vi "WS1050 36 DUT Reliability HD_Cycling_CP CVSweep_Ver1.2.vi"() -> ()   [LabVIEW 2012]
uses:
  WS_VCAP Driver 029/Source/WSVCAP Shell/Type Defs/WSVCAP SHL I2C DUT Mask Mode Enum.ctl
  SubVI/WS105x Run Sequences.ctl
  <vilib>/Utility/file.llb/Read From Spreadsheet File (DBL).vi
panel:
  out "All Data Out":string[](array[string])
  in  "RFFE Slave Address":u8=7 caption="Slave Address" format="0x%02x"
  in  "Reg1_Bit Cntrl":string[](array[string])=["01", "02", "04", "08", "10", "20", "40", "80", "03", "06", "0C", "D8", "33", "66", "CC", "07", "0E", "1C", "38", "70", "E0", "0F", "1E", "3C", "78", "F0", "1F", "3E", "7C", "F8", "3F", "7E", "FC", "7F", "FE", "FD", "FB", "F7", "EF", "DF", "BF", "7F", "FC", "F9", "F3", "E7", "CF", "9F", "3F", "F8", "F1", "E3", "C7", "8F", "1F", "F0", "E1", "C3", "87", "0F", "E0", "C1", "83", "07", "C0", "81", "03", "AA", "55", "00"]
  in  "VPI_Cmd":string[](array[string])=["00", "3B", "00"]
  in  "VPI Name":string[](array[string])=["All_Drivers OFF", "All Drivers ON", "All Drivers OFF2"]
  in  "Tab Control":T1(tab)
  in  "CP with DVA ON":i32(ring) items=["CP HDC 35V", "CP HDC 40.25V", "CP HDC 27.5V", "CP HDC 30.5V", "CP HDC 44V", "CP HDC 50V", "CP HDC 55V", "CP HDC 42.5V", "CP HDC 32V"]
  in  "No of Cmd":i64=2
  in  "Board#":string="BRD5"
  in  "Serial Number":string[][](table)=[["DUT", "SN"], ["DUT1", "1"], ["DUT2", "2"], ["DUT3", "3"], ["DUT4", "4"], ["DUT5", "5"], ["DUT6", "6"], ["DUT7", "7"], ["DUT8", "8"], ["DUT9", "9"], ["DUT10", "10"], ["DUT11", "11"], ["DUT12", "12"], ["DUT13", "13"], ["DUT14", "14"], ["DUT15", "15"], ["DUT16", "16"], ["DUT17", "17"], ["DUT18", "18"], ["DUT19", "19"], ["DUT20", "20"], ["DUT21", "21"], ["DUT22", "22"], ["DUT23", "23"], ["DUT24", "24"], ["DUT25", "25"], ["DUT26", "26"], ["DUT27", "27"], ["DUT28", "28"], ["DUT29", "29"], ["DUT30", "30"], ["DUT31", "31"], ["DUT32", "32"], ["DUT33", "33"], ["DUT34", "34"], ["DUT35", "35"], ["DUT36", "36"]]
  in  "SPI Clock Rate (Hz)":dbl=5000000.0 caption="Cycle Speed" format="%.1p Hz"
  in  "Wafer#":string="T7-EB"
  in  "File Name":string="CYC_WS1050_T7_EB_65C_40V_25DC_BRD5_150911_1"
  in  "TMN DC\\CAP Data Log File Path":path=path "C:/WS1050 36 DUT Data"
  in  "Test Program":string="WS1050 36 DUT HD_Cycling_CP CV Sweep Ver1.2"
  out "Current Date":string="8/28/2014"
  out "Current Time":string="0950"
  in  "Start Date":string="10/21/2014"
  in  "Start Time":string="1542"
  in  "Comment":string="CYC65C40V"
  in  "OK Button":bool
  in  "Calibration":bool
  in  "Verify CP":bool
  in  "CP Setting":i32(ring) items=["CP OFF", "CP ON", "CP 35V", "CP 40V", "DVA ON", "DVA OFF", "REG1 ON", "REG1 OFF", "REG2 ON", "REG2 OFF", "REG3 ON", "REG3 OFF"]
  in  "Set VDD":dbl=3.7 format="%.3g"
  in  "Command":string[](array[string])=["0702013B3B3B", "070201000000", "0702013B0000"]
  in  "Clock Rate (Hz)":dbl=1000000.0 caption="Meas Speed" format="%.1p Hz"
  out "AR  Measurent(Hz)":dbl
  in  "PS1 Source":refnum<visa-resource-name>="GPIB0::5::INSTR"
  in  "Ke2000":refnum<visa-resource-name>="GPIB0::9::INSTR"
  in  "CP to HD/Cycle":i32(ring)=1 items=["CP HDC 35V", "CP HDC 40.25V", "CP HDC 27.5V", "CP HDC 30.5V", "CP HDC 44V", "CP HDC 50V", "CP HDC 55V", "CP HDC 42.5V", "CP HDC 32V"]
  out "Simulate FPGA":bool
  out "Online":bool
  out "AR Cycling(Hz)":dbl=5000000.0
  in  "Ke2400":refnum<visa-resource-name>="GPIB0::3::INSTR"
  in  "Initialize AD7747":bool
  in  "DUT Mask Mode":T2=enum."All"
  out "Activity Log":string="05/19/2014 -- 12:24:35.853::WSVCAP::APP::Application Started\n05/19/2014 -- 12:24:37.606::WSVCAP::WSVCAP SHL::WR I2C-REG:0x0A;MASK:0xFFFFFFFFFFFF;C1 DATA:22:22:22:22:22:22:22:22:22:22:22:22:22:22:22:22;C2 DATA:22:22:22:22:22:22:22:22:22:22:22:22:22:22:22:22;C3 DATA:22:22:22:22:22:22:22:22:22:22:22:22:22:22:22:22\r\n05/19/2014 -- 12:24:37.773::WSVCAP::WSVCAP SHL::WR I2C-ST:0,0,4,1\r\n05/19/2014 -- 12:24:37.903::WSVCAP::WSVCAP SHL::RD I2C-BYTES:4;ADD:0x00;MASK:0xFFFFFFFFFFFF\r\n05/19/2014 -- 12:24:38.045::WSVCAP::WSVCAP SHL::RD I2C:C1 DATA:2:2:2:2:2:2:2:2:2:2:2:2:2:2:2:2|A7:A9:AA:82:82:7F:82:81:82:81:83:82:81:82:82:81|46:36:BB:88:44:A3:E9:2B:32:20:ED:25:BB:3D:68:B|2C:6A:EB:A7:22:56:FE:CC:36:82:D7:B0:3B:48:F9:CC;C2 DATA:2:2:2:2:2:2:2:2:2:2:2:2:2:2:2:2|94:94:94:80:80:80:80:80:81:7E:7E:81:80:7E:80:80|47:33:15:82:62:B:E8:1C:D7:C3:7D:41:7C:B7:4C:2A|C4:B4:AE:8:1E:D1:4E:37:11:C0:6F:63:42:9D:63:B5;C3 DATA:2:2:2:2:2:2:2:2:2:2:2:2:2:2:2:2|95:95:95:81:81:7E:81:80:84:7D:80:83:81:7E:7F:80|AB:C4:14:B5:7B:52:DF:C9:79:5D:5F:30:99:31:1E:F4|6E:5C:F7:A8:C3:EB:7B:EF:33:92:89:77:4D:67:75:DD;STATUS:0:0:4:0\r\n05/19/2014 -- 12:24:38.046::WSVCAP::WSVCAP SHL::WR I2C-REG:0x0A;MASK:0xFFFFFFFFFFFF;C1 DATA:22:22:22:22:22:22:22:22:22:22:22:22:22:22:22:22;C2 DATA:22:22:22:22:22:22:22:22:22:22:22:22:22:22:22:22;C3 DATA:22:22:22:22:22:22:22:22:22:22:22:22:22:22:22:22\r\n05/19/2014 -- 12:24:38.089::WSVCAP::WSVCAP SHL::WR I2C-ST:0,0,4,1\r\n05/19/2014 -- 12:24:38.219::WSVCAP::WSVCAP SHL::RD I2C-BYTES:4;ADD:0x00;MASK:0xFFFFFFFFFFFF\r\n05/19/2014 -- 12:24:38.362::WSVCAP::WSVCAP SHL::RD I2C:C1 DATA:2:2:2:2:2:2:2:2:2:2:2:2:2:2:2:2|A7:AB:AA:82:82:82:83:83:82:82:82:82:7F:82:82:81|4B:32:96:83:3E:61:43:17:25:62:AB:4D:A2:40:2E:5|3C:76:2B:B4:EE:E4:A9:1A:AA:A:26:C7:21:2E:87:5B;C2 DATA:2:2:2:2:2:2:2:2:2:2:2:2:2:2:2:2|94:94:94:80:80:80:80:80:80:7F:80:81:80:80:7F:80|4A:32:19:7D:19:6C:79:46:61:7F:4B:B8:A5:30:F3:14|B4:70:A:8C:9C:DC:43:FA:1E:A:C6:21:A:A9:13:F3;C3 DATA:2:2:2:2:2:2:2:2:2:2:2:2:2:2:2:2|95:97:94:81:80:81:82:81:80:7E:81:84:7F:81:80:80|B2:32:D0:A7:9E:4C:AB:D4:EE:D9:F0:82:B7:91:7:FF|C1:91:B6:3D:D8:E:1B:4F:9F:6A:F1:6C:E7:3F:7:BA;STATUS:0:0:4:0\r\n05/19/2014 -- 12:24:38.364::WSVCAP::WSVCAP SHL::WR I2C-REG:0x0A;MASK:0xFFFFFFFFFFFF;C1 DATA:22:22:22:22:22:22:22:22:22:22:22:22:22:22:22:22;C2 DATA:22:22:22:22:22:22:22:22:22:22:22:22:22:22:22:22;C3 DATA:22:22:22:22:22:22:22:22:22:22:22:22:22:22:22:22\r\n05/19/2014 -- 12:24:38.406::WSVCAP::WSVCAP SHL::WR I2C-ST:0,0,4,1\r\n05/19/2014 -- 12:24:38.536::WSVCAP::WSVCAP SHL::RD I2C-BYTES:4;ADD:0x00;MASK:0xFFFFFFFFFFFF\r\n05/19/2014 -- 12:24:38.678::WSVCAP::WSVCAP SHL::RD I2C:C1 DATA:2:2:2:2:2:2:2:2:2:2:2:2:2:2:2:2|A7:A9:AB:82:82:81:82:82:82:82:82:82:82:82:82:81|46:71:4C:87:43:3D:7F:FC:25:4F:8E:54:97:3E:60:8C|AA:F4:1F:B5:CE:43:1F:36:9:87:9C:78:86:5:B6:8E;C2 DATA:2:2:2:2:2:2:2:2:2:2:2:2:2:2:2:2|94:94:94:80:7F:7F:80:80:80:80:80:81:80:80:80:80|49:36:18:7D:6E:C5:E4:3C:81:2E:41:D3:75:71:E3:72|E8:D3:E6:D1:E0:48:AE:D4:54:D:E8:8E:B4:41:68:4;C3 DATA:2:2:2:2:2:2:2:2:2:2:2:2:2:2:2:2|95:95:95:81:7F:7F:81:81:81:81:81:84:81:81:82:81|B3:F5:90:AB:82:69:7B:93:D0:77:E8:D5:E8:8C:84:E8|B9:AC:EE:2B:B6:71:8F:4A:74:31:56:BB:8A:B7:A0:C8;STATUS:0:0:4:0\r\n05/19/2014 -- 12:24:38.681::WSVCAP::WSVCAP SHL::WR I2C-REG:0x0A;MASK:0xFFFFFFFFFFFF;C1 DATA:22:22:22:22:22:22:22:22:22:22:22:22:22:22:22:22;C2 DATA:22:22:22:22:22:22:22:22:22:22:22:22:22:22:22:22;C3 DATA:22:22:22:22:22:22:22:22:22:22:22:22:22:22:22:22\r\n05/19/2014 -- 12:24:38.723::WSVCAP::WSVCAP SHL::WR I2C-ST:0,0,4,1\r\n05/19/2014 -- 12:24:38.854::WSVCAP::WSVCAP SHL::RD I2C-BYTES:4;ADD:0x00;MASK:0xFFFFFFFFFFFF\r\n05/19/2014 -- 12:24:38.996::WSVCAP::WSVCAP SHL::RD I2C:C1 DATA:2:2:2:2:2:2:2:2:2:2:2:2:2:2:2:2|A7:A9:AA:82:82:7F:83:81:82:81:84:82:7F:82:7F:82|43:FB:E:7F:3C:AD:35:35:26:A2:6C:21:4B:3D:8:6|63:9A:E1:F3:95:32:91:42:90:3C:78:1F:5C:D7:5F:D8;C2 DATA:2:2:2:2:2:2:2:2:2:2:2:2:2:2:2:2|94:94:94:80:80:80:80:80:81:80:7E:81:80:7E:7F:80|48:36:18:7F:5E:3D:69:83:DE:AE:A1:9E:31:AE:BB:96|15:A0:44:17:13:FD:CC:C8:6D:B2:EF:A7:C:C7:3B:F;C3 DATA:2:2:2:2:2:2:2:2:2:2:2:2:2:2:2:2|95:96:94:81:81:7E:82:80:84:80:80:84:7F:7E:7D:82|AD:3B:6D:A9:7C:57:9D:F5:7A:96:23:5C:36:2D:ED:5A|CD:46:DB:3B:C7:BD:70:60:33:B8:B:F7:63:A:51:4D;STATUS:0:0:4:0\r\n05/19/2014 -- 12:24:38.998::WSVCAP::WSVCAP SHL::WR I2C-REG:0x0A;MASK:0xFFFFFFFFFFFF;C1 DATA:22:22:22:22:22:22:22:22:22:22:22:22:22:22:22:22;C2 DATA:22:22:22:22:22:22:22:22:22:22:22:22:22:22:22:22;C3 DATA:22:22:22:22:22:22:22:22:22:22:22:22:22:22:22:22\r\n05/19/2014 -- 12:24:39.040::WSVCAP::WSVCAP SHL::WR I2C-ST:0,0,4,1\r\n05/19/2014 -- 12:24:39.170::WSVCAP::WSVCAP SHL::RD I2C-BYTES:4;ADD:0x00;MASK:0xFFFFFFFFFFFF\r\n05/19/2014 -- 12:24:39.311::WSVCAP::WSVCAP SHL::RD I2C:C1 DATA:2:2:2:2:2:2:2:2:2:2:2:2:2:2:2:2|A7:AA:AB:82:82:81:82:81:82:81:82:82:82:82:7F:82|44:F1:90:87:45:44:C8:2C:2C:F1:FC:1B:94:3B:3C:75|4A:49:95:19:99:73:64:3:23:24:F3:A2:5E:7F:C4:B6;C2 DATA:2:2:2:2:2:2:2:2:2:2:2:2:2:2:2:2|94:94:94:80:80:80:80:7F:80:80:7E:80:80:7E:7F:80|4C:36:17:7D:A8:9F:DE:C7:53:6D:8A:F4:41:A5:C6:E0|90:2E:24:C:D9:22:E4:76:3B:40:1D:53:33:B1:3E:4D;C3 DATA:2:2:2:2:2:2:2:2:2:2:2:2:2:2:2:2|95:97:95:81:81:7F:81:80:80:81:7F:82:81:7E:7D:82|AE:2B:A7:AB:CC:CD:A4:38:FD:17:80:F2:92:2D:45:C4|76:E5:D:B9:AD:B5:BA:8D:28:32:9E:42:B7:20:4A:D9;STATUS:0:0:4:0\r\n05/19/2014 -- 12:24:39.313::WSVCAP::WSVCAP SHL::WR I2C-REG:0x0A;MASK:0xFFFFFFFFFFFF;C1 DATA:22:22:22:22:22:22:22:22:22:22:22:22:22:22:22:22;C2 DATA:22:22:22:22:22:22:22:22:22:22:22:22:22:22:22:22;C3 DATA:22:22:22:22:22:22:22:22:22:22:22:22:22:22:22:22\r\n05/19/2014 -- 12:24:39.355::WSVCAP::WSVCAP SHL::WR I2C-ST:0,0,4,1\r\n05/19/2014 -- 12:24:39.486::WSVCAP::WSVCAP SHL::RD I2C-BYTES:4;ADD:0x00;MASK:0xFFFFFFFFFFFF\r\n05/19/2014 -- 12:24:39.628::WSVCAP::WSVCAP SHL::RD I2C:C1 DATA:2:2:2:2:2:2:2:2:2:2:2:2:2:2:2:2|A7:A9:AA:82:82:82:83:82:82:82:82:82:7F:82:7F:82|47:18:E4:87:3E:E7:6:65:25:92:37:38:A8:3E:89:85|7C:A7:7:2B:A3:7A:EC:EF:89:ED:F4:D3:D8:BC:3A:F5;C2 DATA:2:2:2:2:2:2:2:2:2:2:2:2:2:2:2:2|94:94:94:80:7F:80:80:7F:81:80:7E:80:80:80:81:80|49:37:17:80:76:25:6A:F8:DF:55:97:4D:B8:5B:2B:B1|13:E3:9A:3E:1A:2D:4F:B6:DB:E9:61:FA:8B:D6:9:CC;C3 DATA:2:2:2:2:2:2:2:2:2:2:2:2:2:2:2:2|95:95:95:81:7F:80:82:81:84:80:7F:81:80:81:7F:82|AF:93:3B:AF:5B:11:82:E4:7E:C3:2D:72:9:96:D9:A|DB:96:F2:10:5F:64:9A:C6:98:12:27:7D:10:D3:20:D9;STATUS:0:0:4:0\r\n05/19/2014 -- 12:24:40.132::WSVCAP::WSVCAP SHL::CLOSE\r\n"
  in  "C1 Cap DAC":u8=128 caption="B Data In" format="0x%02x"
  in  "C2 Cap DAC":u8=128 caption="B Data In" format="0x%02x"
  in  "C3 Cap DAC":u8=128 caption="B Data In" format="0x%02x"
  out "IDD Brd(uA)":string
  in  "Repeat Meas(s)":u32=900
  in  "Real No. From\nLookup Table":bool
  in  "Control Panel":T3={"Verify Socket"=FALSE, "HD/CYC"=FALSE, "E-CAL"=FALSE, "DVA"=FALSE, "VPI"=TRUE, "VSA"=TRUE, "HS"=FALSE}
  out "Verify Socket":bool
  out "HD/CYC":bool
  out "E-CAL":bool
  out "DVA":bool
  out "VPI":bool
  out "VSA":bool
  out "HS":bool
  in  "Lot#":string="WS1050"
  out "AD7747 Values":string[][](table)
  in  "Freq(Hz)":string="12K"
  in  "Reset P/S":bool
  in  "Test Sequences":i32(ring) items=["C1_C2_C3", "C2_C1_C3", "C3_C2_C1"]
  in  "WS1050/51":bool=TRUE
  in  "% Duty Cycle":string="25"
  in  "Cmd To HD":string="0702013B3B3B"
  in  "Post CMd Delay":dbl[](array[numeric])=[1.7e-05, 5.4e-05, 1.8e-05] min=0.0 max=0.5 format="%#.0p s"
  in  "Cmin/Act":bool=TRUE
  in  "CP VPI":i32(ring) items=["CP HDC 35V", "CP HDC 40.25V", "CP HDC 27.5V", "CP HDC 30.5V", "CP HDC 44V", "CP HDC 50V", "CP HDC 55V", "CP HDC 42.5V", "CP HDC 32V"]
  in  "WS105x Run Sequences":T4
  out "CAP_C1":string[][](table)
  out "NOM IDD OFF(uA)":string
  out "CAP_C2":string[][](table)
  out "CAP_C3":string[][](table)
  in  "Set HD/Cycle \nto Complete":u64=5000000000
  out "No of HD/Cycle\nCompleted":u64
  out "Cycle Count":u64 min=1 max=4 step=1
  out "Loop \ncompleted":i32=1
  out "Previous Time":string="12:20:26 PM"
  out "STATUS":string="Idle...."
  out "Total Delta C2(pF)":string[](array[string])
  out "Total Delta C1(pF)":string[](array[string])
  out "Total Delta C3(pF)":string[](array[string])
  out "RB Reg for HD":string[](array[string])
  out "RB Reg for HD/Cycle":string[](array[string])
  out "VPI C2":string[][](table)
  out "VPI C3":string[][](table)
  out "NOM IDD ON (uA)":string
  out "IDD_HD/CYC (uA)":string="164.601255E+0"
  in  "stop During HD/Cycles":bool
  in  "stop":bool
  out "IDD Stdby(uA)":string="2.606990E+0"
  out "VPI C1":string[][](table)
  in  "DeltaC Target Setting(pF)":dbl=7.375
  out "VSA_V1":string[][](table)
  out "VSA_V2":string[][](table)
  out "VSA_V3":string[][](table)
  in  "VSA Voltage(V)":dbl[](array[numeric])=[-10.0, 0.0, 10.0]
  in  "DC_Temp":i32=65
  in  "HD/CYC Temp":i32=65
  in  "Time All ON (s)":u32=120
  in  "Time All OFF (s)":u32=120
  in  "HD_DC (Min)":u64=259200
  out "LPs Count":i32
  in  "X Repeat":i32=100
  out "No LPs to RP":i32
  out "Run Loops":i32=1
  out "% Delta C_T0":string[][](array[string])
  out "% Delta C":string[][](array[string])
  out "EFuse RB T0":string[](array[string])
  out "Current EFuse Read back":string[](array[string])
  out "EFuse Readback Status":bool[](array[boolean])
  out "error out":errorcluster
  in  "error in (no error)":errorcluster
  in  "HD RP":dbl=60.0
  in  "Cycle RP":dbl=10000.0
  out "Min Plot_1":dbl[][](graph) caption="(Y) Multi Plot 2"
  out "Min Plot_2":dbl[][](graph) caption="(Y) Multi Plot 2"
  out "Min Plot_3":dbl[][](graph) caption="(Y) Multi Plot 2"
  in  "Plot Delta Cmin":bool=TRUE
  in  "Plot":T5(ring)
  in  "Bank C1":i32(ring) items=["C1", "C2", "C3", "D_C1", "D_C2", "D_C3"]
  in  "Bank C2":i32(ring)=1 items=["C1", "C2", "C3", "D_C1", "D_C2", "D_C3"]
  in  "Bank C3":i32(ring)=2 items=["C1", "C2", "C3", "D_C1", "D_C2", "D_C3"]
  in  "Manual Setting\nFor RP CP CV":i64[](array[numeric])=[0, 100000, 5000000]
  in  "CP CV \nSweep":bool=TRUE
  out "CP CV Sweep C1":dbl[][](graph) caption="(Y) Multi Plot 2"
  out "CP CV Sweep C2":dbl[][](graph) caption="(Y) Multi Plot 2"
  out "CP CV Sweep C3":dbl[][](graph) caption="(Y) Multi Plot 2"
  out "LP CP Voltage":string
  in  "Auto\nMan":bool
  in  "Start":i64
  in  "Stop":i64
  in  "Step":i64
  out "RP for CP CV":i64[](array[numeric])
  out "CP to Run":dbl[](array[numeric])
  # "Company:  WiSpry Inc\n20 Fairbanks Ste 198 Irvine CA 92618\n\nAuthor:  Andy V Tran\nCreated:  10/06/2015\nLabVIEW 2012 Pro\nTest Program:  WS1050 36 DUT Reliability HD_Cycling CP CV Sweep ver1.1\nFPGA: WS_VCAP Driver 029"
  # "Note for HD Duty Cycle:\n1.  Set time to start HD_DC (Min), default is 259200 (6 months) \n2.  Set Time for Duty Cycle ON/OFF, default setting is 2 minutes\n3.  No of Loops to RP = 3600s/(Time ALL ON(s) + Time ALL + OFF(s))\n4.  Set X Repeat = no of runs, default is 100 runs\n5.  Set TTF Completed to stop the test.\n\nVer 1.1:\n1.  Set CP voltage measure F1, F2 and B1"
  # "Minutes"
  # "X1000"
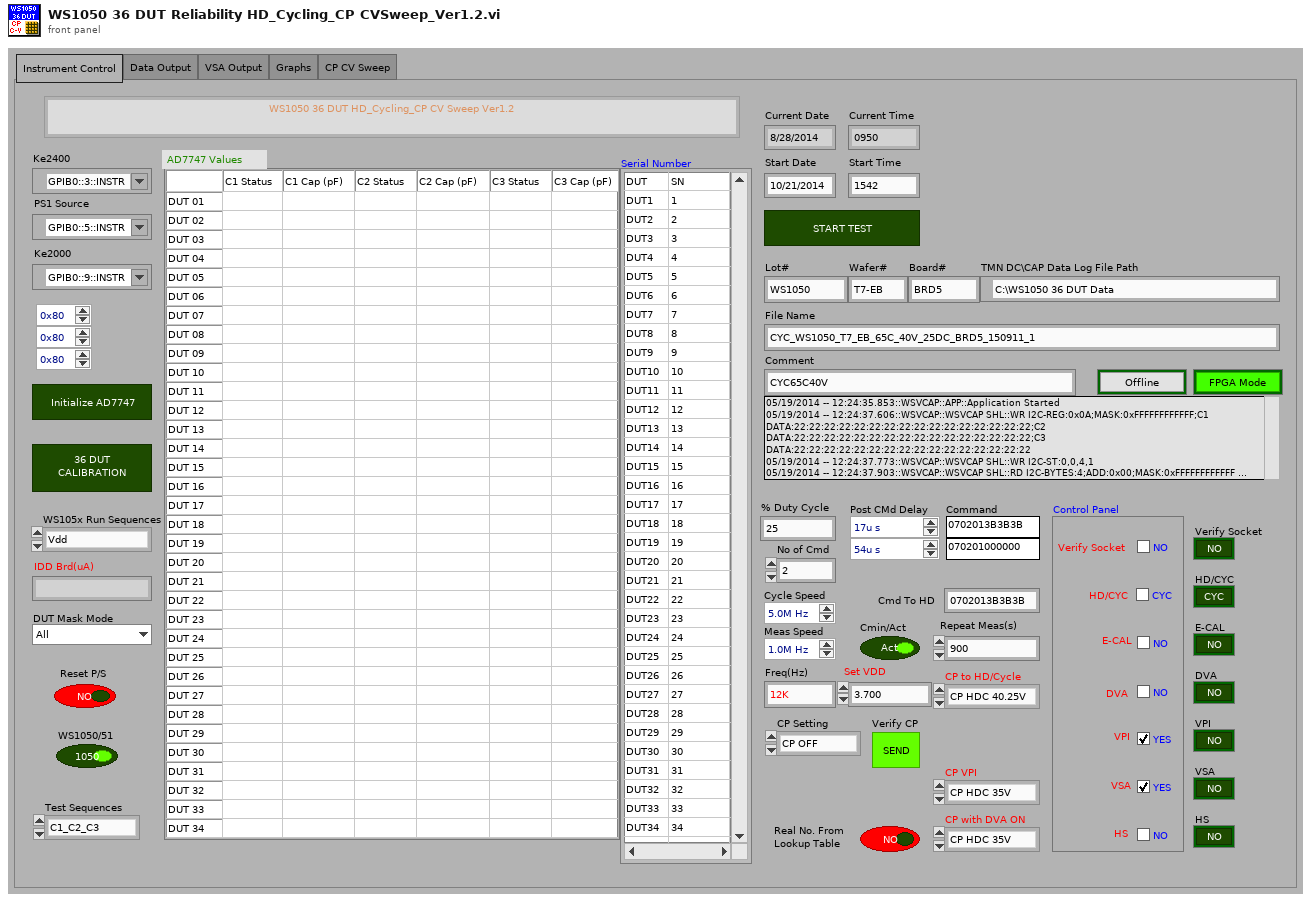
[diagram p1: front panel]
types:
  T1 = enum32{"Instrument Control", "Data Output", "VSA Output", "Graphs", "CP CV Sweep"}
  T2 = typedef "WSVCAP SHL I2C DUT Mask Mode Enum.ctl" = enum16{"Custom", "C1", "C2", "C3", "All"}
  T3 = cluster{"Verify Socket":bool, "HD/CYC":bool, "E-CAL":bool, "DVA":bool, "VPI":bool, "VSA":bool, "HS":bool}
  T4 = typedef "WS105x Run Sequences.ctl" = enum16{"Vdd", "Select CP", "Idd", "Stress", "Meas CAP", "VPI", "VSA", "HS CHK", "Save Data", "CPV SWPT", "CPV Data", "Idle..."}
  T5 = enum16{"ALL DUTs", "DUT 01", "DUT 02", "DUT 03", "DUT 04", "DUT 05", "DUT 06", "DUT 07", "DUT 08", "DUT 09", "DUT 10", "DUT 11", "DUT 12", "DUT 13", "DUT 14", "DUT 15", "DUT 16", "DUT 17", "DUT 18", "DUT 19", "DUT 20", "DUT 21", "DUT 22", "DUT 23", "DUT 24", "DUT 25", "DUT 26", "DUT 27", "DUT 28", "DUT 29", "DUT 30", "DUT 31", "DUT 32", "DUT 33", "DUT 34", "DUT 35", "DUT 36"}
  T6 = typedef "WSVCAP SHL Core System Cluster.ctl" = cluster{"Settings":T7, "FPGA Resource":tag, "Online":bool, "I2C Wait Ticks":u32, "SPI Wait Ticks":u32, "RFFE Wait Ticks":u32}
  T7 = typedef "WSVCAP SHL I2C Settings Cluster.ctl" = cluster{"FPGA Resource Name":string, "I2C Slave Address":u8, "I2C Clock Rate (Hz)":dbl, "SPI Clock Rate (Hz)":dbl, "RFFE Slave Address":u8, "RFFE Clock Rate (Hz)":dbl, "Simulate FPGA":bool, "C1 Cap DAC Default":u8, "C2 Cap DAC Default":u8, "C3 Cap DAC Default":u8}
  T8 = enum16{"Idle...", "Voltage 1", "Voltage 2", "Voltage 3"}[]
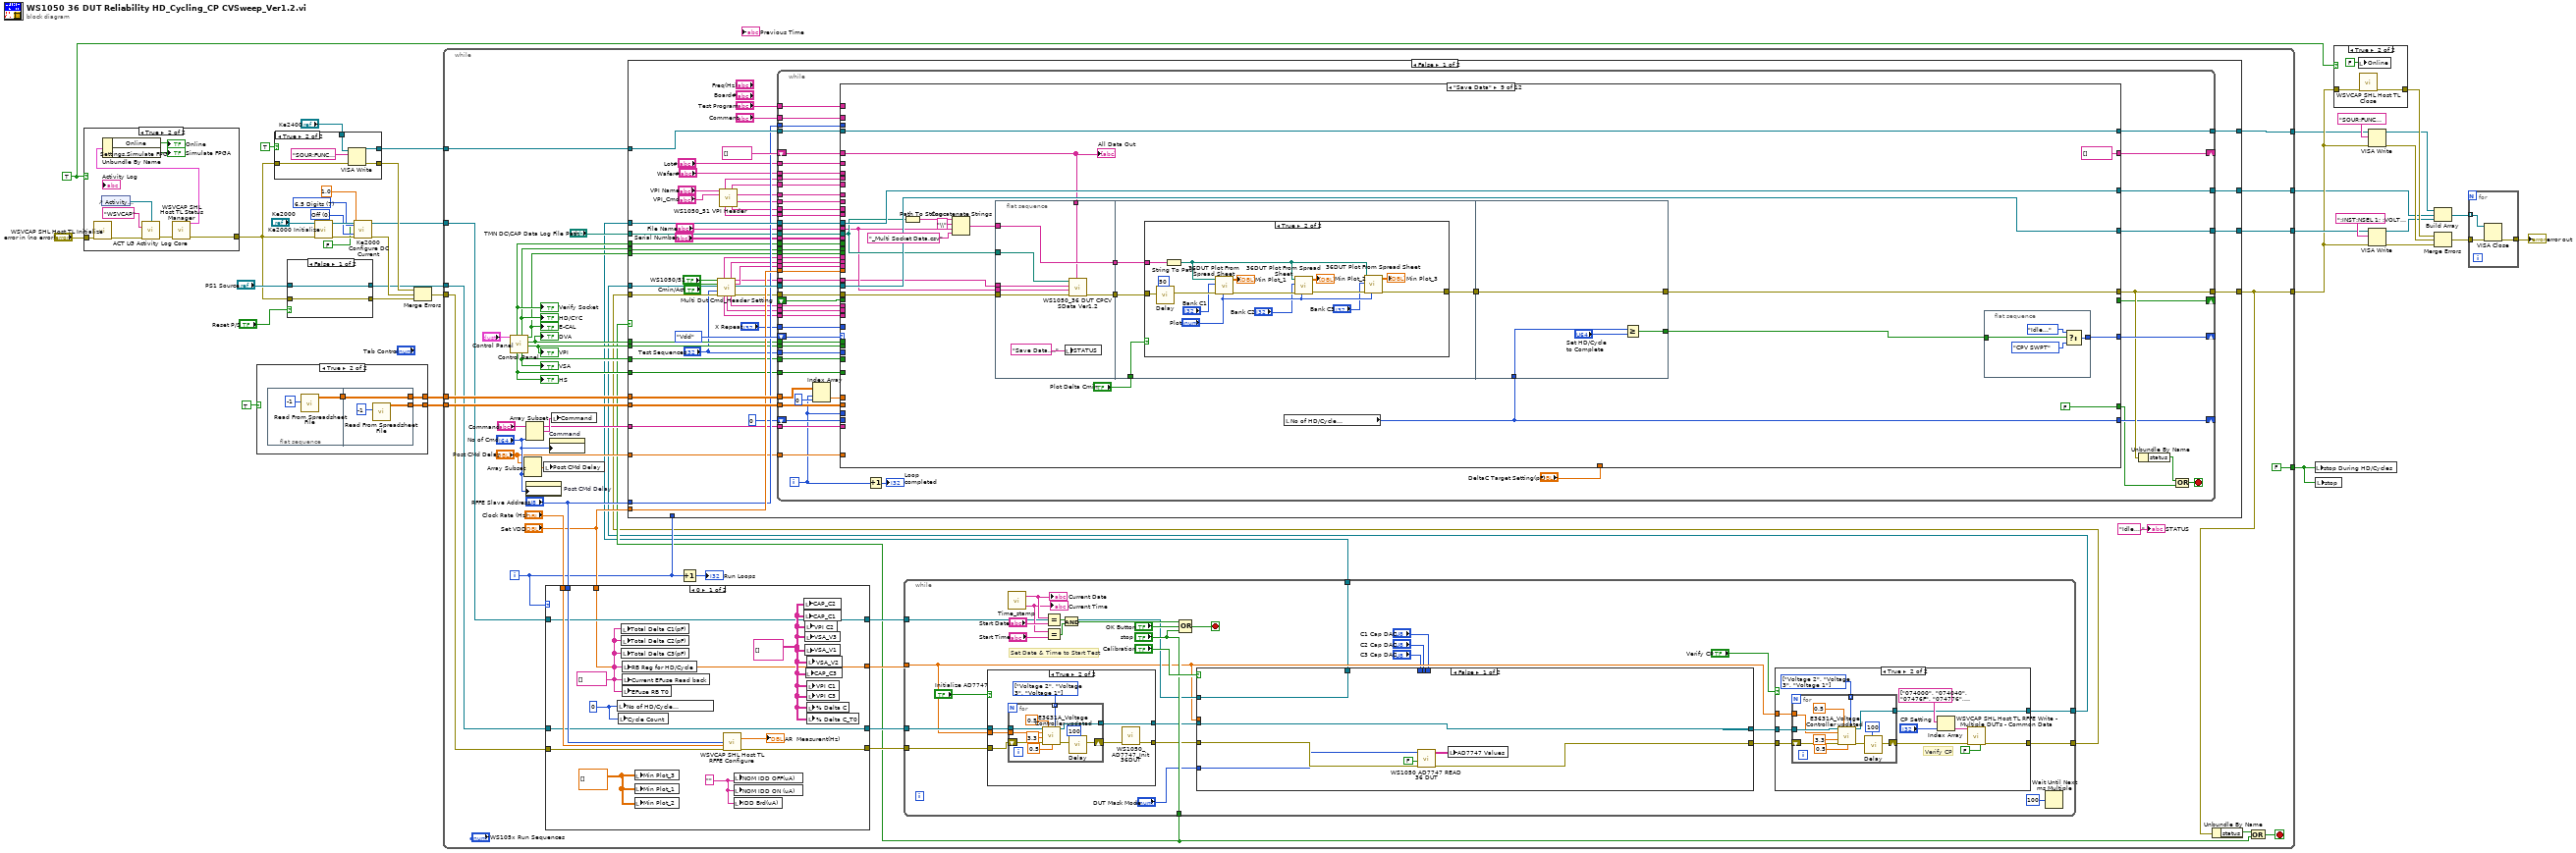
[diagram p0: block diagram]
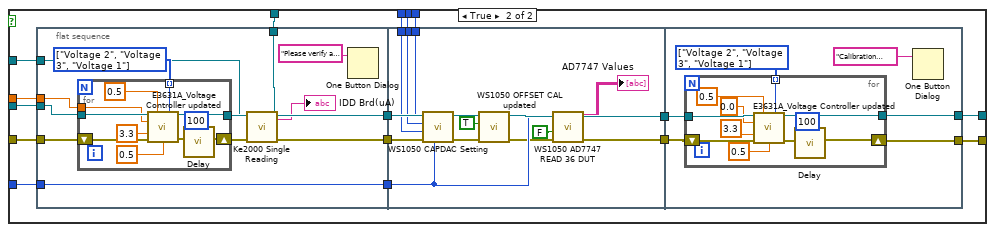
[diagram p5: hidden frame]
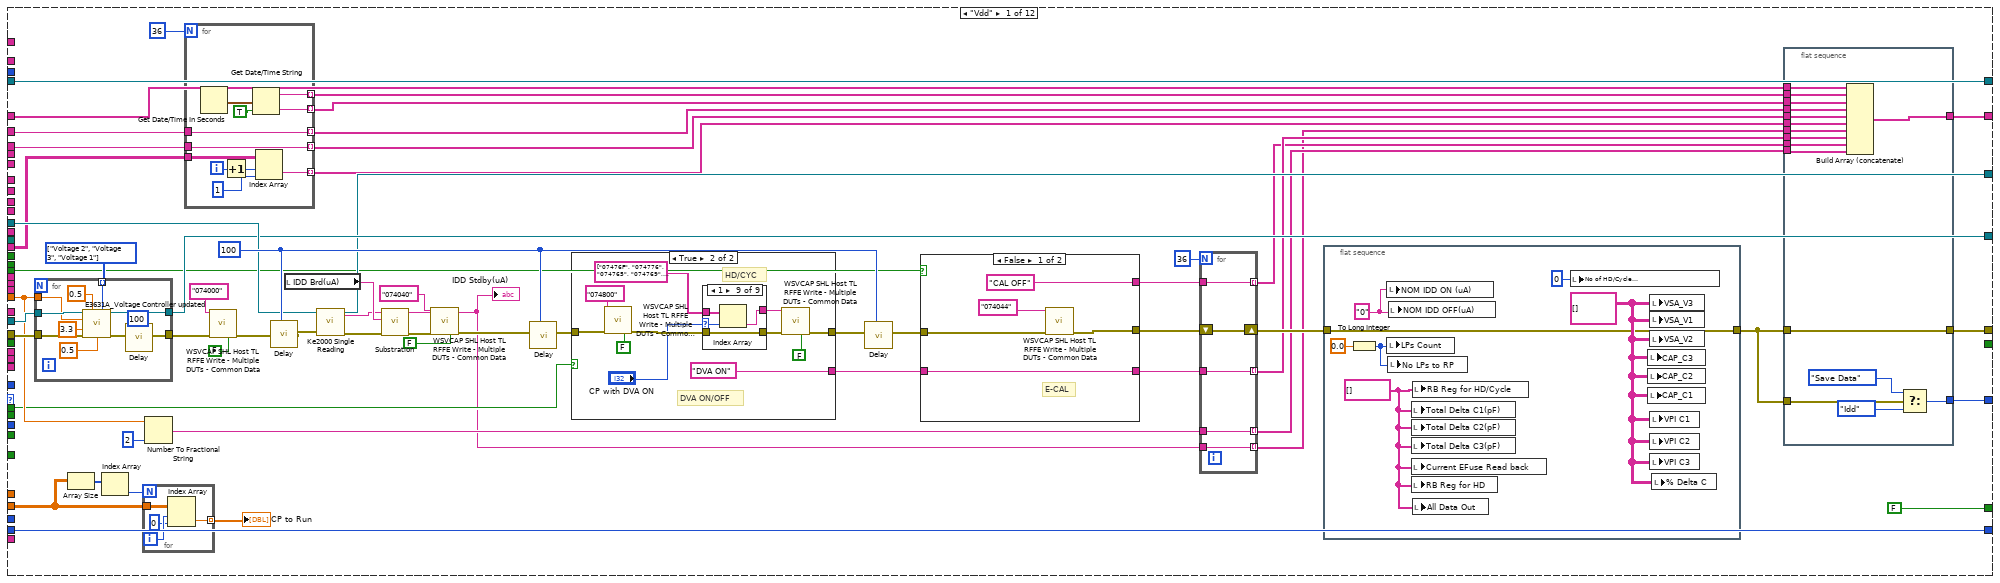
[diagram p6: hidden frame]
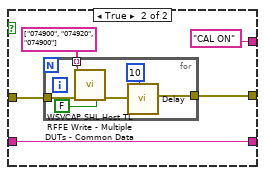
[diagram p7: hidden frame]
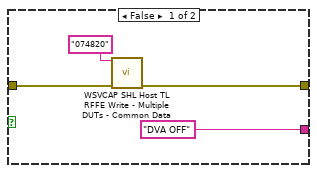
[diagram p8: hidden frame]
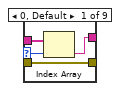
[diagram p9: hidden frame]
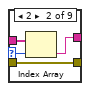
[diagram p10: hidden frame]
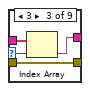
[diagram p11: hidden frame]
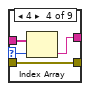
[diagram p12: hidden frame]
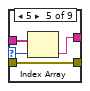
[diagram p13: hidden frame]
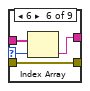
[diagram p14: hidden frame]
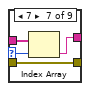
[diagram p15: hidden frame]
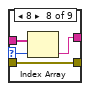
[diagram p16: hidden frame]
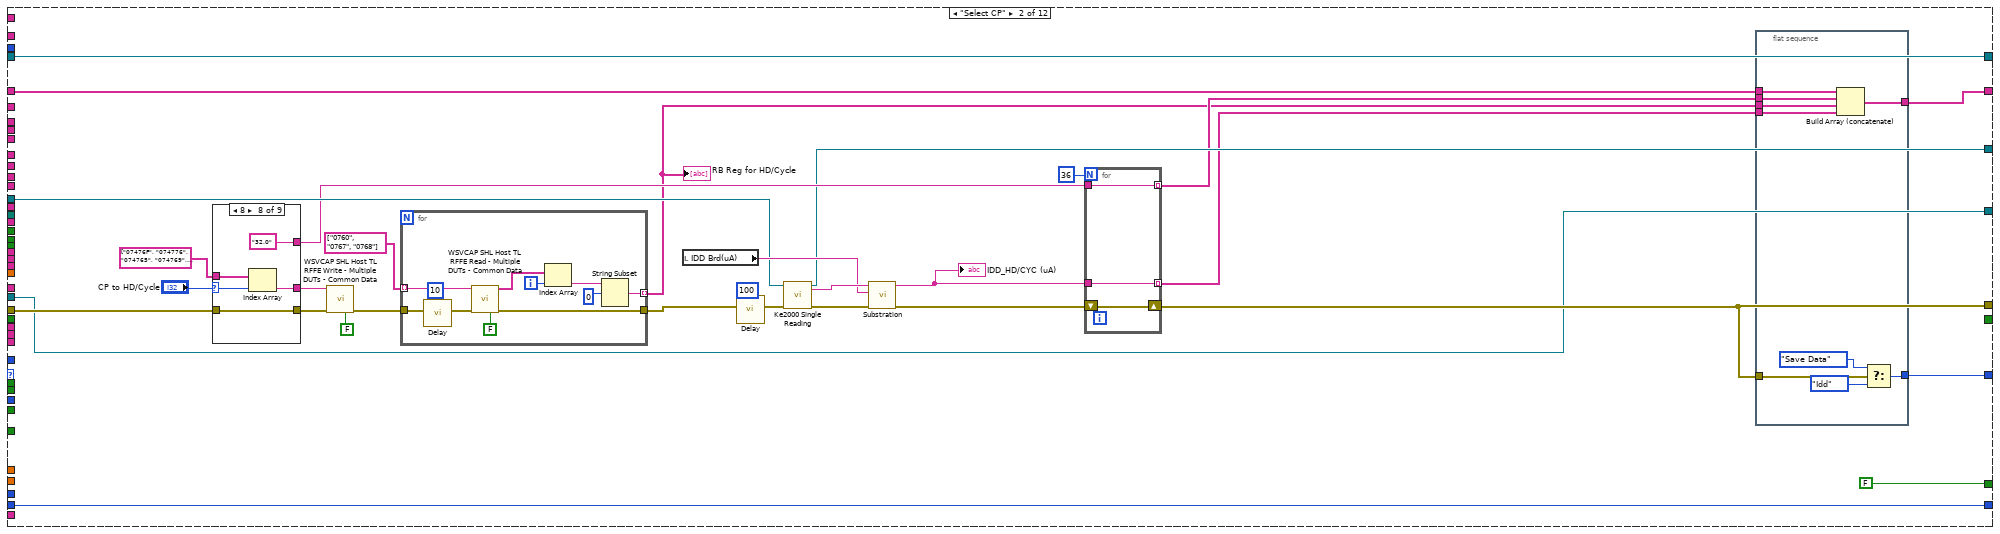
[diagram p17: hidden frame]
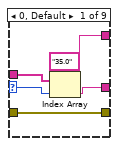
[diagram p18: hidden frame]
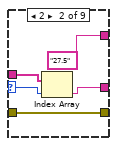
[diagram p19: hidden frame]
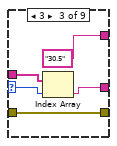
[diagram p20: hidden frame]
diagram:
  w14 = TRUE
  w34 = u16 0 items=["Off", "Moving Filter", "Repeating Filter"] ("Digital Filter (0: Off)")
  w35 = u16 7 items=["3.5 Digits"=4, "4.5 Digits"=5, "5.5 Digits"=6, "6.5 Digits"=7] ("Resolution (7: 6.5 digits)")
  n1 = case shown="True" w14 {
    tunnel: "error in (no error)" -> [w40 w41]
    tunnel: [w40 w48] -> w25
    frame False {
    }
    frame True {
      n2 = call "WSVCAP SHL Host TL Initialize.vi"("error in"=w41) -> ("error out"=w42:errorcluster)  [unwired: 13 in, 1 out]
      n3 = control-ref of="Activity Log"() -> (w44:refnum<vi>)
      n4 = call "ACT LG Activity Log Core.vi"("Display Ref"=w44, "Source"="WSVCAP", "Error In (no error)"=w42) -> ("Error Out"=w43:errorcluster)  [unwired: 11 in, 1 out]
      n5 = call "WSVCAP SHL Host TL Status Manager.vi"("error in"=w43) -> ("System Out"=w49:T6, "error out"=w48:errorcluster)  [unwired: 13 in]
      n6 = Unbundle By Name(w49) -> ("Online"=→"Online":bool, "Settings.Simulate FPGA"=→"Simulate FPGA":bool)
    }
  }
  n7 = case shown="True" TRUE {
    tunnel: [_ w52] -> w19
    tunnel: [_ w50] -> w18
    frame False {
    }
    frame True {
      n8 = flat-sequence {
        tunnel: [w53] -> w51
        tunnel: [w57] -> w52
        tunnel: w51 -> [w57]
        tunnel: [w55] -> w50
        frame #0 {
          n9 = call-poly <vilib>:"Read From Spreadsheet File.vi"("number of rows (all:-1)"=-1) -> ("all rows"=w53:dbl[][])  [unwired: 6 in, 4 out]
        }
        frame #1 {
          n10 = call-poly <vilib>:"Read From Spreadsheet File.vi"("number of rows (all:-1)"=-1) -> ("all rows"=w55:dbl[][])  [unwired: 6 in, 4 out]
        }
      }
    }
  }
  n11 = case shown="True" TRUE {
    tunnel: w25 -> [w58 w63]
    tunnel: [w59 w62] -> w17
    tunnel: [w58 w61] -> w28
    tunnel: "Ke2400" -> [w59 w60]
    frame False {
    }
    frame True {
      n12 = VISA Write(VISA resource name=w60, write buffer="SOUR:FUNC VOLT;VOLT:MODE FIX;RANG 100;LEV 0.0;:SENS:FUNC \"CURR\";CURR:PROT 60E-3;RANG 100E-3;:OUTP ON", error in (no error)=w63) -> (VISA resource name out=w62:refnum<visa-resource-name>, error out=w61:errorcluster)  [unwired: 1 out]
    }
  }
  n13 = case shown="False" "Reset P/S" {
    tunnel: "PS1 Source" -> [w65 w72]
    tunnel: [w65 w70] -> w15
    tunnel: w25 -> [w66 w68]
    tunnel: [w66 w67] -> w24
    frame False {
    }
    frame True {
      n14 = call "Agilent 3631A Initialize.vi"("error in (no error)"=w68, "Default"=FALSE ("Reset? (T: Yes)"), "Reset"=TRUE ("ID Query? (T: Yes)"), "VISA resource name"=w72) -> ("error out"=w67:errorcluster, "VISA resource name out"=w70:refnum<visa-resource-name>)  [unwired: 6 in]
    }
  }
  n15 = call "Ke2000 Initialize.vi"("error in (no error)"=w25, "VISA resource name"="Ke2000") -> ("error out"=w36:errorcluster, "VISA resource name out"=w37:refnum<visa-resource-name>)  [unwired: 8 in]
  n16 = call "Ke2000 Configure DC Current.vi"("Resolution (7: 6.5 digits)"=w35, "Digital Filter (0: Off)"=w34, "Auto Range? (T: Auto)"=FALSE, "error in"=w36, "Custom Range (0 A)"=1.0, "VISA resource name"=w37) -> ("error out"=w26:errorcluster, "VISA resource name out"=w16:refnum<visa-resource-name>)  [unwired: 4 in]
  n17 = Merge Errors(w28, w26, w24) -> (w20:errorcluster)
  n18 = while {
    tunnel: w20 -> [w76]
    tunnel: w19 -> [w109]
    tunnel: w18 -> [w110]
    tunnel: w17 -> [w82]
    tunnel: w16 -> [w74]
    tunnel: w15 -> [w85]
    tunnel: [w112] -> w12
    tunnel: [w108] -> w13
    tunnel: [w107] -> w4
    tunnel: [w106] -> w10
    tunnel: [FALSE ("stop During HD/Cycles")] -> w9
    i -> [w79]
    stop <- w113 stop-if-true
    n19 = call "Control Panel.vi"("Control Panel"="Control Panel") -> ("VPI"=w100:bool, "DVA"=w101:bool, "E-CAL"=w102:bool, "VSA"=w99:bool, "HD/CYC"=w103:bool, "HS"=w98:bool, "Verify Socket"=w104:bool)  [unwired: 3 in, 1 out]
    "Verify Socket" <- w104
    "E-CAL" <- w102
    "VPI" <- w100
    "VSA" <- w99
    "HS" <- w98
    "HD/CYC" <- w103
    "DVA" <- w101
    n20 = Array Subset(array="Post CMd Delay", length="No of Cmd") -> (w96:dbl[])  [unwired: 1 in]
    n21 = Array Subset(array="Command", length="No of Cmd") -> (w97:string[])  [unwired: 1 in]
    n22 = property on="Post CMd Delay" class="Arr (strict)"("Number of Rows"="No of Cmd") -> ()  [unwired: 2 in, 2 out]
    n23 = local write "Post CMd Delay"(w96) -> ()
    n24 = case shown="0" w79 {
      tunnel: [w125 w130] -> w86
      tunnel: w76 -> [w119 w130]
      tunnel: "RFFE Slave Address" -> [w118 _]
      tunnel: "Clock Rate (Hz)" -> [w117 _]
      tunnel: w85 -> [w116 w129]
      tunnel: [w116 w129] -> w84
      tunnel: [w115 w128] -> w83
      tunnel: w74 -> [w115 w128]
      tunnel: "Set VDD" -> [w114 w127]
      tunnel: [w114 w127] -> w80
      frame 0 {
        w121 = dbl[][] []
        w120 = "" ("uA")
        w122 = string[][] []
        w123 = string[] [] ("EFuse Read back")
        w126 = u64 0 ("No of HD/Cycle\nCompleted")
        n25 = local write "No of HD/Cycle\nCompleted"(w126) -> ()
        n26 = local write "Cycle Count"(w126) -> ()
        n27 = local write "Total Delta C1(pF)"(w123) -> ()
        n28 = local write "Total Delta C2(pF)"(w123) -> ()
        n29 = local write "Total Delta C3(pF)"(w123) -> ()
        n30 = local write "RB Reg for HD/Cycle"(w123) -> ()
        n31 = local write "Current EFuse Read back"(w123) -> ()
        n32 = local write "EFuse RB T0"(w123) -> ()
        n33 = local write "Min Plot_3"(w121) -> ()
        n34 = local write "Min Plot_1"(w121) -> ()
        n35 = local write "Min Plot_2"(w121) -> ()
        n36 = call "WSVCAP SHL Host TL RFFE Configure.vi"("RFFE Slave Address"=w118, "Clock Rate (Hz)"=w117, "error in"=w119) -> ("Actual Rate (Hz)"=→"AR  Measurent(Hz)":dbl, "error out"=w125:errorcluster)  [unwired: 11 in]
        n37 = local write "NOM IDD OFF(uA)"(w120) -> ()
        n38 = local write "NOM IDD ON (uA)"(w120) -> ()
        n39 = local write "IDD Brd(uA)"(w120) -> ()
        n40 = local write "CAP_C2"(w122) -> ()
        n41 = local write "CAP_C1"(w122) -> ()
        n42 = local write "VPI C2"(w122) -> ()
        n43 = local write "VSA_V3"(w122) -> ()
        n44 = local write "VSA_V1"(w122) -> ()
        n45 = local write "CAP_C3"(w122) -> ()
        n46 = local write "VSA_V2"(w122) -> ()
        n47 = local write "VPI C1"(w122) -> ()
        n48 = local write "VPI C3"(w122) -> ()
        n49 = local write "% Delta C"(w122) -> ()
        n50 = local write "% Delta C_T0"(w122) -> ()
      }
      frame 1, Default {
      }
    }
    n51 = property on="Command" class="Arr (strict)"("Number of Rows"="No of Cmd") -> ()  [unwired: 2 in, 2 out]
    n52 = local write "Command"(w97) -> ()
    n53 = Increment(x=w79) -> (x+1=→"Run Loops":i32)
    n54 = while {
      tunnel: ["stop"] -> w78
      tunnel: w86 -> [w145]
      tunnel: [w132] -> w75
      tunnel: w84 -> [w144]
      tunnel: w83 -> [w140]
      tunnel: [w141] -> w77
      tunnel: w80 -> [w138]
      tunnel: [w131] -> w73
      stop <- w152 stop-if-true
      # "Set Date & Time to Start Test"
      n55 = case shown="True" "Initialize AD7747" {
        tunnel: w145 -> [w161 w167]
        tunnel: [w161 w164] -> w139
        tunnel: w144 -> [w160 w165]
        tunnel: w138 -> [_ w163]
        tunnel: [w160 w162] -> w133
        frame False {
        }
        frame True {
          w168 = T8 [enum."Voltage 2", enum."Voltage 3", enum."Voltage 1"] items=["Idle...", "Voltage 1", "Voltage 2", "Voltage 3"]
          n56 = for {
            tunnel: w165 -> [w178]
            tunnel: w168 -> [w176] mode=indexing
            tunnel: [w175] -> w162
            shift-right: [w172] -> w166
            shift-left: w167 -> [w179]
            tunnel: w163 -> [w169]
            n57 = call "E3631A_Voltage Controller updated.vi"("VISA resource name"=w178, "I_VDD(A)"=0.5, "Channel Controller"=w176, "Voltage 1"=w169, "Voltage 2"=3.3, "error in (no error)"=w179, "I_3.3V (A)"=0.5) -> ("VISA resource name out"=w175:refnum<visa-resource-name>, "error out"=w171:errorcluster)  [unwired: 7 in]
            n58 = call "Delay.vi"("milliseconds to wait"=u32 100, "error in (no error)"=w171) -> ("error out"=w172:errorcluster)  [unwired: 9 in]
          }
          n59 = call "WS1050_AD7747_Init 36DUT.vi"("error in"=w166) -> ("error out"=w164:errorcluster)  [unwired: 10 in]
        }
      }
      n60 = call "Time_stamp.vi"() -> ("date/time string"=w157:string, "date string"=w159:string)  [unwired: 2 in]
      "Current Date" <- w159
      "Current Time" <- w157
      n61 = Equal?(x=w159, y="Start Date") -> (x = y?=w155:bool)
      n62 = Equal?(x=w157, y="Start Time") -> (x = y?=w154:bool)
      n63 = And(x=w155, y=w154) -> (x .and. y?=w151:bool)
      n64 = Compound Arithmetic op=OR(w151, "OK Button", "stop") -> (w152:bool)
      n65 = case shown="False" "Calibration" {
        tunnel: w139 -> [w210 w226]
        tunnel: [w205 w223] -> w134
        tunnel: w133 -> [w209 w222]
        tunnel: "DUT Mask Mode" -> [w208 w218]
        tunnel: [w209 w217] -> w142
        tunnel: w140 -> [w204 w216]
        tunnel: w138 -> [_ w215]
        tunnel: "C1 Cap DAC" -> [_ w214]
        tunnel: "C2 Cap DAC" -> [_ w213]
        tunnel: "C3 Cap DAC" -> [_ w212]
        tunnel: [w204 w211] -> w131
        frame False {
          n66 = call "WS1050 AD7747 READ 36 DUT.vi"("error in"=w210, "Log (T)"=FALSE, "DUT Mask Mode (All)"=w208) -> ("error out"=w205:errorcluster, "AD7747 Values"=w206:string[][])  [unwired: 7 in]
          n67 = local write "AD7747 Values"(w206) -> ()
        }
        frame True {
          n68 = flat-sequence {
            tunnel: w226 -> [w236]
            tunnel: [w231] -> w225
            tunnel: w222 -> [w235]
            tunnel: [w234] -> w221
            tunnel: w218 -> [w233]
            tunnel: [w233] -> w219
            tunnel: w216 -> [w229]
            tunnel: w215 -> [w228]
            tunnel: [w227] -> w211
            tunnel: w225 -> [w261]
            tunnel: [w260] -> w224
            tunnel: w221 -> [w259]
            tunnel: [w259] -> w220
            tunnel: w219 -> [w258]
            tunnel: w214 -> [w254]
            tunnel: w213 -> [w253]
            tunnel: w212 -> [w252]
            tunnel: w224 -> [w263]
            tunnel: [w266] -> w223
            tunnel: w220 -> [w265]
            tunnel: [w262] -> w217
            frame #0 {
              w237 = T8 [enum."Voltage 2", enum."Voltage 3", enum."Voltage 1"] items=["Idle...", "Voltage 1", "Voltage 2", "Voltage 3"]
              n69 = for {
                tunnel: w235 -> [w248]
                tunnel: w237 -> [w246] mode=indexing
                tunnel: [w245] -> w234
                shift-right: [w243] -> w230
                shift-left: w236 -> [w249]
                tunnel: w228 -> [w239]
                n70 = call "E3631A_Voltage Controller updated.vi"("VISA resource name"=w248, "I_VDD(A)"=0.5, "Channel Controller"=w246, "Voltage 1"=w239, "Voltage 2"=3.3, "error in (no error)"=w249, "I_3.3V (A)"=0.5) -> ("VISA resource name out"=w245:refnum<visa-resource-name>, "error out"=w242:errorcluster)  [unwired: 7 in]
                n71 = call "Delay.vi"("milliseconds to wait"=u32 100, "error in (no error)"=w242) -> ("error out"=w243:errorcluster)  [unwired: 9 in]
              }
              n72 = call "Ke2000 Single Reading.vi"("error in (no error)"=w230, "VISA resource name"=w229) -> ("error out"=w231:errorcluster, "VISA resource name out"=w227:refnum<visa-resource-name>, "uA"=→"IDD Brd(uA)":string)  [unwired: 5 in, 2 out]
              n73 = One Button Dialog(message="Please verify all sockets should be empty...") -> ()  [unwired: 1 in, 1 out]
            }
            frame #1 {
              n74 = call "WS1050 CAPDAC Setting.vi"("DUT Mask Mode (All)"=w258, "error in"=w261, "C3 Cap DAC"=w252, "C2 Cap DAC"=w253, "C1 Cap DAC"=w254) -> ("error out"=w256:errorcluster)  [unwired: 6 in]
              n75 = call "WS1050 OFFSET CAL updated.vi"("error in"=w256, "OFFSET CAL"=TRUE ("Read?")) -> ("error out"=w255:errorcluster)  [unwired: 9 in]
              n76 = call "WS1050 AD7747 READ 36 DUT.vi"("error in"=w255, "Log (T)"=FALSE, "DUT Mask Mode (All)"=w258) -> ("error out"=w260:errorcluster, "AD7747 Values"=→"AD7747 Values":string[][])  [unwired: 7 in]
            }
            frame #2 {
              w264 = T8 [enum."Voltage 2", enum."Voltage 3", enum."Voltage 1"] items=["Idle...", "Voltage 1", "Voltage 2", "Voltage 3"]
              n77 = for {
                tunnel: w265 -> [w278]
                tunnel: w264 -> [w275] mode=indexing
                tunnel: [w274] -> w262
                shift-right: [w270] -> w266
                shift-left: w263 -> [w276]
                n78 = call "E3631A_Voltage Controller updated.vi"("VISA resource name"=w278, "I_VDD(A)"=0.5, "Channel Controller"=w275, "Voltage 1"=0.0, "Voltage 2"=3.3, "error in (no error)"=w276, "I_3.3V (A)"=0.5) -> ("VISA resource name out"=w274:refnum<visa-resource-name>, "error out"=w269:errorcluster)  [unwired: 7 in]
                n79 = call "Delay.vi"("milliseconds to wait"=u32 100, "error in (no error)"=w269) -> ("error out"=w270:errorcluster)  [unwired: 9 in]
              }
              n80 = One Button Dialog(message="Calibration Completed....") -> ()  [unwired: 1 in, 1 out]
            }
          }
        }
      }
      n81 = case shown="True" "Verify CP" {
        tunnel: [w180 w185] -> w132
        tunnel: w142 -> [w181 w188]
        tunnel: [w181 w186] -> w141
        tunnel: w134 -> [w180 w184]
        tunnel: w138 -> [_ w182]
        frame False {
        }
        frame True {
          w189 = T8 [enum."Voltage 2", enum."Voltage 3", enum."Voltage 1"] items=["Idle...", "Voltage 1", "Voltage 2", "Voltage 3"]
          # "Verify CP"
          n82 = for {
            tunnel: w188 -> [w202]
            tunnel: w189 -> [w200] mode=indexing
            shift-right: [w198] -> w187
            shift-left: w184 -> [w203]
            tunnel: [w196] -> w186
            tunnel: w182 -> [w193]
            n83 = call "E3631A_Voltage Controller updated.vi"("VISA resource name"=w202, "I_VDD(A)"=0.5, "Channel Controller"=w200, "Voltage 1"=w193, "Voltage 2"=3.3, "error in (no error)"=w203, "I_3.3V (A)"=0.5) -> ("VISA resource name out"=w196:refnum<visa-resource-name>, "error out"=w199:errorcluster)  [unwired: 7 in]
            n84 = call "Delay.vi"("milliseconds to wait"=u32 100, "error in (no error)"=w199) -> ("error out"=w198:errorcluster)  [unwired: 9 in]
          }
          n85 = Index Array(array=string[] ["074000", "074040", "07476F", "074776", "074800", "074820", "07413B", "074100", "07423B", "074200", "07433B", "074300"], index="CP Setting") -> (element=w190:string)
          n86 = call "WSVCAP SHL Host TL RFFE Write - Multiple DUTs - Common Data.vi"("Data Out"=w190, "error in"=w187, "Log (T)"=FALSE) -> ("error out"=w185:errorcluster)  [unwired: 12 in]
        }
      }
      n87 = Wait Until Next ms Multiple(millisecond multiple=u32 100) -> ()  [unwired: 1 out]
    }
    n88 = case shown="False" w78 {
      tunnel: w79 -> [_ _]
      tunnel: w75 -> [w303 w1896]
      tunnel: [w326 w1896] -> w112
      tunnel: w73 -> [w328 w1894]
      tunnel: w77 -> [w327 w1895]
      tunnel: w110 -> [w325 _]
      tunnel: w109 -> [w324 _]
      tunnel: [w323 w1895] -> w108
      tunnel: w82 -> [w320 w1893]
      tunnel: "Set VDD" -> [w322 _]
      tunnel: "RFFE Slave Address" -> [w317 _]
      tunnel: [w321 w1894] -> w107
      tunnel: [w319 w1893] -> w106
      tunnel: w104 -> [w316 _]
      tunnel: w103 -> [w315 _]
      tunnel: w102 -> [w314 _]
      tunnel: w101 -> [w313 _]
      tunnel: w100 -> [w312 _]
      tunnel: w99 -> [w311 _]
      tunnel: w98 -> [w310 _]
      tunnel: "Command" -> [w308 _]
      tunnel: "Post CMd Delay" -> [w309 _]
      tunnel: "TMN DC\\CAP Data Log File Path" -> [w286 _]
      frame False {
        n89 = call "Multi Dut Cmd_Header Setting.vi"("WS1050/51"="WS1050/51", "Cmin/Act"="Cmin/Act", "Test Seq"="Test Sequences", "error in (no error)"=w303) -> ("Name 1"=w300:string[], "Name 2"=w299:string[], "Name Header"=w279:string[], "Name 3"=w298:string[], "Cmd 1"=w297:string[], "Extended Cmd"=w296:string[], "Cmd 2"=w295:string[], "error out"=w302:errorcluster)  [unwired: 2 in, 2 out]
        n90 = call "WS1050_51 VPI Header.vi"("VPI Name"="VPI Name", "VPI_Cmd"="VPI_Cmd") -> ("VPI_1"=w292:string[], "VPI_2"=w291:string[], "VPI_3"=w290:string[], "Cmd_3"=w289:string[], "Cmd_1"=w287:string[], "Cmd_2"=w288:string[])  [unwired: 6 in, 2 out]
        n91 = while {
          shift-right: [w387] -> _
          shift-left: WS105x_Run_Sequences."Vdd" ("WS105x Run Sequences") -> [w388]
          tunnel: w302 -> [w386]
          tunnel: w328 -> [w385]
          tunnel: w327 -> [w384]
          tunnel: [w360] -> w326
          tunnel: w325 -> [w383]
          tunnel: w324 -> [w381]
          tunnel: [w379] -> w323
          tunnel: w322 -> [w378]
          tunnel: [w377] -> w321
          tunnel: w320 -> [w376]
          tunnel: [w375] -> w319
          shift-right: [w374] -> _
          shift-left: string[] [] -> [w373]
          tunnel: w316 -> [w372]
          tunnel: w317 -> [w371]
          tunnel: w315 -> [w370]
          tunnel: w314 -> [w369]
          tunnel: w313 -> [w368]
          tunnel: w312 -> [w367]
          tunnel: w311 -> [w366]
          tunnel: w310 -> [w365]
          tunnel: w309 -> [w364]
          tunnel: w308 -> [w363]
          tunnel: "X Repeat" -> [w362]
          shift-right: [w358] -> _
          shift-left: u64 0 -> [w361]
          tunnel: "Test Sequences" -> [w357]
          tunnel: w300 -> [w356]
          tunnel: w299 -> [w355]
          tunnel: w298 -> [w354]
          tunnel: w297 -> [w353]
          tunnel: w296 -> [w352]
          tunnel: w295 -> [w351]
          tunnel: w292 -> [w349]
          tunnel: w291 -> [w348]
          tunnel: w290 -> [w347]
          tunnel: w289 -> [w346]
          tunnel: w288 -> [w344]
          tunnel: w287 -> [w345]
          tunnel: w286 -> [w343]
          tunnel: "Lot#" -> [w342]
          tunnel: "Wafer#" -> [w341]
          tunnel: "File Name" -> [w340]
          tunnel: "Serial Number" -> [w339]
          shift-right: [w336] -> _
          shift-left: _ -> [w335]
          tunnel: "Test Program" -> [w334]
          tunnel: "Comment" -> [w333]
          tunnel: w279 -> [w332]
          i -> [w337]
          stop <- w359 stop-if-true
          n92 = Index Array(array=w381, index (row)=w337, index (col)=0 ("disabled index (col)")) -> (element=w380:dbl)
          n93 = case shown="\"Save Data\"" w388 {
            tunnel: [w424 w584 w685 w734 w1007 w1346 w1566 w1716 w1776 w1817 w1873 w1888] -> w387
            tunnel: w386 -> [w428 w588 w686 w744 w990 w1361 w1570 w1718 w1779 w1825 w1872 w1884]
            tunnel: w385 -> [w427 w586 w687 w731 w1011 w1347 w1558 w1712 w1772 w1820 w1875 w1886]
            tunnel: w384 -> [w426 w576 w682 w732 w1010 w1348 w1560 w1711 w1773 w1819 w1874 w1883]
            tunnel: [w398 w579 w677 w729 w997 w1344 w1564 w1714 w1775 w1822 w1872 w1884] -> w360
            tunnel: w383 -> [w423 _ _ _ _ _ _ _ _ _ _ _]
            tunnel: w380 -> [_ _ _ w743 _ _ _ _ _ _ _ _]
            tunnel: w378 -> [w412 _ _ _ _ _ _ _ _ _ _ _]
            tunnel: [w422 w576 w682 w732 w1010 w1347 w1559 w1711 w1773 w1819 w1874 w1883] -> w379
            tunnel: [w421 w578 w684 w731 w1011 w1348 w1558 w1712 w1772 w1820 w1875 w1886] -> w377
            tunnel: w376 -> [w420 w580 w683 w733 w1012 w1353 w1569 w1713 w1774 w1821 w1877 w1882]
            tunnel: [w420 w580 w683 w733 w1012 w1353 w1562 w1713 w1774 w1821 w1877 w1882] -> w375
            tunnel: [w400 w570 w669 w716 w999 w1339 w1551 w1706 string[] [] _ _ _] -> w374
            tunnel: w373 -> [w390 w574 w672 w720 w1006 w1343 w1555 w1709 w1764 _ _ _]
            tunnel: w372 -> [_ _ _ w742 _ _ _ _ _ _ _ _]
            tunnel: w337 -> [_ _ _ w741 w994 _ _ w1725 _ _ _ _]
            tunnel: w371 -> [_ _ _ w740 w991 _ _ _ _ _ _ _]
            tunnel: w370 -> [_ _ _ w739 _ _ _ _ _ _ _ _]
            tunnel: w369 -> [w410 _ _ _ _ _ _ _ _ _ _ _]
            tunnel: w368 -> [w409 _ _ _ _ _ w1557 _ _ _ _ _]
            tunnel: w367 -> [_ _ _ _ _ w1354 _ _ _ _ _ _]
            tunnel: w366 -> [_ _ _ _ _ _ w1563 _ _ _ _ _]
            tunnel: w365 -> [_ _ _ _ _ _ _ w1726 _ _ _ _]
            tunnel: w364 -> [_ _ _ w737 _ _ _ _ _ _ _ _]
            tunnel: w363 -> [_ _ _ w736 _ _ _ _ _ _ _ _]
            tunnel: w362 -> [_ _ _ w735 _ _ _ _ _ _ _ _]
            tunnel: [w394 w575 w674 w722 w995 w1349 w1561 w1710 w1760 w1823 w1876 w1887] -> w358
            tunnel: w361 -> [w394 w575 w674 w723 w995 w1349 w1561 w1710 _ w1823 w1876 w1887]
            tunnel: w357 -> [_ _ _ _ w1032 _ _ _ _ _ _ _]
            tunnel: w356 -> [_ _ _ _ w1031 _ _ _ _ _ _ _]
            tunnel: w355 -> [_ _ _ _ w1030 _ _ _ _ _ _ _]
            tunnel: w354 -> [_ _ _ _ w1029 _ _ _ _ _ _ _]
            tunnel: w353 -> [_ _ _ _ w1028 _ _ _ _ _ _ _]
            tunnel: w352 -> [_ _ _ _ w1016 _ _ _ _ _ _ _]
            tunnel: w351 -> [_ _ _ _ w1015 _ _ _ _ _ _ _]
            tunnel: "DeltaC Target Setting(pF)" -> [_ _ _ _ w1008 _ _ _ _ _ _ _]
            tunnel: w349 -> [_ _ _ _ _ w1360 _ _ _ _ _ _]
            tunnel: w348 -> [_ _ _ _ _ w1359 _ _ _ _ _ _]
            tunnel: w347 -> [_ _ _ _ _ w1358 _ _ _ _ _ _]
            tunnel: w346 -> [_ _ _ _ _ w1355 _ _ _ _ _ _]
            tunnel: w345 -> [_ _ _ _ _ w1357 _ _ _ _ _ _]
            tunnel: w344 -> [_ _ _ _ _ w1356 _ _ _ _ _ _]
            tunnel: w343 -> [_ _ _ _ _ _ _ w1724 w1767 _ _ _]
            tunnel: w342 -> [w397 _ _ _ _ _ _ w1723 _ _ _ _]
            tunnel: w341 -> [w396 _ _ _ _ _ _ w1722 _ _ _ _]
            tunnel: w340 -> [_ _ _ _ _ _ _ w1721 w1763 w1824 _ _]
            tunnel: w339 -> [w395 _ _ _ _ _ _ w1720 _ _ _ _]
            tunnel: [FALSE ("true") FALSE ("true") FALSE ("true") FALSE ("true") FALSE ("true") FALSE ("true") FALSE ("true") FALSE ("true") FALSE ("true") FALSE ("true") _ TRUE ("true")] -> w330
            tunnel: [_ _ _ w721 _ _ _ _ _ _ _ _] -> w336
            tunnel: w335 -> [_ _ _ _ w996 _ _ _ _ _ _ _]
            tunnel: w334 -> [_ _ _ _ _ _ _ _ _ _ _ _]
            tunnel: w333 -> [_ _ _ _ _ _ _ _ _ _ _ _]
            tunnel: w332 -> [_ _ _ _ _ _ _ _ w1762 _ _ _]
            frame "Vdd" {
              w440 = u32 100 ("milliseconds to wait")
              w429 = T8 [enum."Voltage 2", enum."Voltage 3", enum."Voltage 1"] items=["Idle...", "Voltage 1", "Voltage 2", "Voltage 3"]
              n94 = for {
                tunnel: w428 -> [w568]
                tunnel: w426 -> [w567]
                tunnel: w429 -> [w565] mode=indexing
                tunnel: [w561] -> w431
                tunnel: [w564] -> w422
                tunnel: w412 -> [w558]
                n95 = call "E3631A_Voltage Controller updated.vi"("VISA resource name"=w567, "I_VDD(A)"=0.5, "Channel Controller"=w565, "Voltage 1"=w558, "Voltage 2"=3.3, "error in (no error)"=w568, "I_3.3V (A)"=0.5) -> ("VISA resource name out"=w564:refnum<visa-resource-name>, "error out"=w562:errorcluster)  [unwired: 7 in]
                n96 = call "Delay.vi"("milliseconds to wait"=u32 100, "error in (no error)"=w562) -> ("error out"=w561:errorcluster)  [unwired: 9 in]
              }
              n97 = Array Size(array=w423) -> (size(s)=w445:i32[])
              n98 = Index Array(array=w445) -> (element=w446:i32)  [unwired: 1 in]
              n99 = for {
                N: w446 -> [_]
                tunnel: w423 -> [w489]
                tunnel: [w488] -> w447 mode=indexing
                i -> [w490]
                n100 = Index Array(array=w489, index (row)=w490, index (col)=0 ("disabled index (col)")) -> (element=w488:dbl)
              }
              "CP to Run" <- w447
              n101 = Number To Fractional String(number=w412, precision (6)=i16 2) -> (F-format string=w411:string)  [unwired: 2 in]
              n102 = for {
                N: 36 -> [_]
                tunnel: w395 -> [w458]
                tunnel: [w456] -> w404 mode=indexing
                tunnel: [w451] -> w408 mode=indexing
                tunnel: [w450] -> w407 mode=indexing
                tunnel: [w449] -> w406 mode=indexing
                tunnel: [w448] -> w405 mode=indexing
                tunnel: w397 -> [w449]
                tunnel: w396 -> [w448]
                i -> [w455]
                n103 = Get Date/Time In Seconds() -> (seconds since 1Jan1904=w453:timestamp)
                n104 = Increment(x=w455) -> (x+1=w454:i32)
                n105 = Get Date/Time String(seconds (now)=w453, want seconds? (F)=TRUE) -> (date string=w451:string, time string=w450:string)  [unwired: 1 in]
                n106 = Index Array(array=w458, index (row)=w454, index (col)=1 ("disabled index (col)")) -> (element=w456:string)
              }
              n107 = call "WSVCAP SHL Host TL RFFE Write - Multiple DUTs - Common Data.vi"("Data Out"="074000", "error in"=w431, "Log (T)"=FALSE) -> ("error out"=w430:errorcluster)  [unwired: 12 in]
              n108 = call "Delay.vi"("milliseconds to wait"=w440, "error in (no error)"=w430) -> ("error out"=w432:errorcluster)  [unwired: 9 in]
              n109 = local read "IDD Brd(uA)"() -> (w439:string)
              n110 = call "Ke2000 Single Reading.vi"("error in (no error)"=w432, "VISA resource name"=w427) -> ("error out"=w438:errorcluster, "VISA resource name out"=w421:refnum<visa-resource-name>, "uA"=w437:string)  [unwired: 5 in, 2 out]
              n111 = call "Substration.vi"("error in (no error)"=w438, "Input2"=w439, "Input1"=w437) -> ("error out"=w443:errorcluster, "In1 - In2"=w392:string)  [unwired: 7 in]
              "IDD Stdby(uA)" <- w392
              n112 = call "WSVCAP SHL Host TL RFFE Write - Multiple DUTs - Common Data.vi"("Data Out"="074040", "error in"=w443, "Log (T)"=FALSE) -> ("error out"=w444:errorcluster)  [unwired: 12 in]
              n113 = call "Delay.vi"("milliseconds to wait"=w440, "error in (no error)"=w444) -> ("error out"=w434:errorcluster)  [unwired: 9 in]
              n114 = case shown="True" w409 {
                tunnel: w434 -> [w510 w519]
                tunnel: [w509 w517] -> w435
                tunnel: ["DVA OFF" ("Data Out") "DVA ON" ("Data Out")] -> w415
                frame False {
                  n115 = call "WSVCAP SHL Host TL RFFE Write - Multiple DUTs - Common Data.vi"("Data Out"="074820", "error in"=w510) -> ("error out"=w509:errorcluster)  [unwired: 13 in]
                }
                frame True {
                  # "DVA ON/OFF"
                  # "HD/CYC"
                  n116 = call "WSVCAP SHL Host TL RFFE Write - Multiple DUTs - Common Data.vi"("Data Out"="074800", "error in"=w519, "Log (T)"=FALSE) -> ("error out"=w515:errorcluster)  [unwired: 12 in]
                  n117 = case shown="1" "CP with DVA ON" {
                    selector: "CP with DVA ON" -> [w525 w529 w533 w537 w541 w545 w549 w553 w557]
                    tunnel: [w524 w528 w532 w536 w540 w544 w548 w552 w555] -> w512
                    tunnel: [w523 w527 w531 w535 w539 w543 w547 w551 w556] -> w514
                    tunnel: w515 -> [w523 w527 w531 w535 w539 w543 w547 w551 w556]
                    tunnel: string[] ["07476F", "074776", "074765", "074769", "07477B", "07477C", "07477D", "074779", "07476B"] -> [w522 w526 w530 w534 w538 w542 w546 w550 w554]
                    frame 0, Default {
                      n118 = Index Array(array=w522, index=w525) -> (element=w524:string)
                    }
                    frame 2 {
                      n119 = Index Array(array=w526, index=w529) -> (element=w528:string)
                    }
                    frame 3 {
                      n120 = Index Array(array=w530, index=w533) -> (element=w532:string)
                    }
                    frame 4 {
                      n121 = Index Array(array=w534, index=w537) -> (element=w536:string)
                    }
                    frame 5 {
                      n122 = Index Array(array=w538, index=w541) -> (element=w540:string)
                    }
                    frame 6 {
                      n123 = Index Array(array=w542, index=w545) -> (element=w544:string)
                    }
                    frame 7 {
                      n124 = Index Array(array=w546, index=w549) -> (element=w548:string)
                    }
                    frame 8 {
                      n125 = Index Array(array=w550, index=w553) -> (element=w552:string)
                    }
                    frame 1 {
                      n126 = Index Array(array=w554, index=w557) -> (element=w555:string)
                    }
                  }
                  n127 = call "WSVCAP SHL Host TL RFFE Write - Multiple DUTs - Common Data.vi"("Data Out"=w512, "error in"=w514, "Log (T)"=FALSE) -> ("error out"=w517:errorcluster)  [unwired: 12 in]
                }
              }
              n128 = call "Delay.vi"("milliseconds to wait"=w440, "error in (no error)"=w435) -> ("error out"=w425:errorcluster)  [unwired: 9 in]
              n129 = case shown="False" w410 {
                tunnel: w425 -> [w495 w498]
                tunnel: [w492 w497] -> w419
                tunnel: ["CAL OFF" ("Data Out") "CAL ON" ("Data Out")] -> w416
                tunnel: w415 -> [w491 w496]
                tunnel: [w491 w496] -> w414
                frame False {
                  # "E-CAL"
                  n130 = call "WSVCAP SHL Host TL RFFE Write - Multiple DUTs - Common Data.vi"("Data Out"="074044", "error in"=w495) -> ("error out"=w492:errorcluster)  [unwired: 13 in]
                }
                frame True {
                  n131 = for {
                    tunnel: string[] ["074900", "074920", "074900"] -> [w506] mode=indexing
                    tunnel: w498 -> [w503]
                    tunnel: [w502] -> w497
                    n132 = call "WSVCAP SHL Host TL RFFE Write - Multiple DUTs - Common Data.vi"("Data Out"=w506, "error in"=w503, "Log (T)"=FALSE) -> ("error out"=w505:errorcluster)  [unwired: 12 in]
                    n133 = call "Delay.vi"("milliseconds to wait"=u32 10, "error in (no error)"=w505) -> ("error out"=w502:errorcluster)  [unwired: 9 in]
                  }
                }
              }
              n134 = for {
                N: 36 -> [_]
                tunnel: w416 -> [w462]
                tunnel: [w462] -> w402 mode=indexing
                shift-right: [w463] -> w418
                shift-left: w419 -> [w463]
                tunnel: [w461] -> w403 mode=indexing
                tunnel: w414 -> [w461]
                tunnel: w411 -> [w460]
                tunnel: [w460] -> w401 mode=indexing
                tunnel: w392 -> [w459]
                tunnel: [w459] -> w391 mode=indexing
              }
              n135 = flat-sequence {
                tunnel: [w466] -> w399
                tunnel: w418 -> [w466]
                frame #0 {
                  w468 = "0" ("NOM IDD OFF(uA)")
                  w464 = string[] []
                  w469 = string[][] []
                  n136 = To Long Integer(number=0.0 ("No of Loops to RP")) -> (32bit integer=w467:i32)
                  n137 = local write "NOM IDD ON (uA)"(w468) -> ()
                  n138 = local write "LPs Count"(w467) -> ()
                  n139 = local write "No LPs to RP"(w467) -> ()
                  n140 = local write "NOM IDD OFF(uA)"(w468) -> ()
                  n141 = local write "Total Delta C1(pF)"(w464) -> ()
                  n142 = local write "Total Delta C2(pF)"(w464) -> ()
                  n143 = local write "Total Delta C3(pF)"(w464) -> ()
                  n144 = local write "Current EFuse Read back"(w464) -> ()
                  n145 = local write "RB Reg for HD"(w464) -> ()
                  n146 = local write "RB Reg for HD/Cycle"(w464) -> ()
                  n147 = local write "All Data Out"(w464) -> ()
                  n148 = local write "No of HD/Cycle\nCompleted"(u64 0 ("No of HD/Cycle\nCompleted")) -> ()
                  n149 = local write "CAP_C3"(w469) -> ()
                  n150 = local write "CAP_C2"(w469) -> ()
                  n151 = local write "CAP_C1"(w469) -> ()
                  n152 = local write "VSA_V3"(w469) -> ()
                  n153 = local write "VSA_V1"(w469) -> ()
                  n154 = local write "VSA_V2"(w469) -> ()
                  n155 = local write "VPI C1"(w469) -> ()
                  n156 = local write "VPI C2"(w469) -> ()
                  n157 = local write "VPI C3"(w469) -> ()
                  n158 = local write "% Delta C"(w469) -> ()
                }
              }
              n159 = flat-sequence {
                tunnel: w399 -> [w485]
                tunnel: [w484] -> w424
                tunnel: w390 -> [w482]
                tunnel: w408 -> [w481]
                tunnel: w407 -> [w480]
                tunnel: w406 -> [w479]
                tunnel: w405 -> [w478]
                tunnel: w404 -> [w477]
                tunnel: w403 -> [w472]
                tunnel: w402 -> [w473]
                tunnel: w401 -> [w474]
                tunnel: [w476] -> w400
                tunnel: w399 -> [w475]
                tunnel: [w475] -> w398
                tunnel: w391 -> [w471]
                frame #0 {
                  n160 = Build Array (concatenate)(w482, w481, w480, w479, w478, w477, w471, w472, w473, w474) -> (w476:string[])
                  n161 = Select(t=WS105x_Run_Sequences."Save Data" ("WS105x Run Sequences"), s=w485, f=WS105x_Run_Sequences."Idd" ("WS105x Run Sequences")) -> (s? t:f=w484:T4)
                }
              }
            }
            frame "Select CP" {
              n162 = case shown="8" "CP to HD/Cycle" {
                selector: "CP to HD/Cycle" -> [w615 w620 w625 w630 w635 w640 w645 w650 w654]
                tunnel: string[] ["07476F", "074776", "074765", "074769", "07477B", "07477C", "07477D", "074779", "07476B"] -> [w616 w621 w626 w631 w636 w641 w646 w651 w656]
                tunnel: [w614 w619 w624 w629 w634 w639 w644 w649 w655] -> w585
                tunnel: ["35.0" ("Data Out") "27.5" ("Data Out") "30.5" ("Data Out") "44.0" ("Data Out") "50.0" ("Data Out") "55.0" ("Data Out") "42.5" ("Data Out") "32.0" ("Data Out") "40.25" ("Data Out")] -> w581
                tunnel: [w612 w617 w622 w627 w632 w637 w642 w647 w652] -> w587
                tunnel: w588 -> [w612 w617 w622 w627 w632 w637 w642 w647 w652]
                frame 0, Default {
                  n163 = Index Array(array=w616, index=w615) -> (element=w614:string)
                }
                frame 2 {
                  n164 = Index Array(array=w621, index=w620) -> (element=w619:string)
                }
                frame 3 {
                  n165 = Index Array(array=w626, index=w625) -> (element=w624:string)
                }
                frame 4 {
                  n166 = Index Array(array=w631, index=w630) -> (element=w629:string)
                }
                frame 5 {
                  n167 = Index Array(array=w636, index=w635) -> (element=w634:string)
                }
                frame 6 {
                  n168 = Index Array(array=w641, index=w640) -> (element=w639:string)
                }
                frame 7 {
                  n169 = Index Array(array=w646, index=w645) -> (element=w644:string)
                }
                frame 8 {
                  n170 = Index Array(array=w651, index=w650) -> (element=w649:string)
                }
                frame 1 {
                  n171 = Index Array(array=w656, index=w654) -> (element=w655:string)
                }
              }
              n172 = call "WSVCAP SHL Host TL RFFE Write - Multiple DUTs - Common Data.vi"("Data Out"=w585, "error in"=w587, "Log (T)"=FALSE) -> ("error out"=w598:errorcluster)  [unwired: 12 in]
              n173 = for {
                tunnel: string[] ["0760", "0767", "0768"] -> [w665] mode=indexing
                tunnel: [w661] -> w572 mode=indexing
                tunnel: w598 -> [w659]
                tunnel: [w658] -> w597
                i -> [w664]
                n174 = call "Delay.vi"("milliseconds to wait"=u32 10, "error in (no error)"=w659) -> ("error out"=w666:errorcluster)  [unwired: 9 in]
                n175 = call "WSVCAP SHL Host TL RFFE Read - Multiple DUTs - Common Data.vi"("Data Out"=w665, "error in"=w666, "Log (T)"=FALSE) -> ("RFFE Data In"=w663:string[], "error out"=w658:errorcluster)  [unwired: 11 in]
                n176 = Index Array(array=w663, index=w664) -> (element=w660:string)
                n177 = String Subset(string=w660, offset (0)=0) -> (substring=w661:string)  [unwired: 1 in]
              }
              "RB Reg for HD/Cycle" <- w572
              n178 = local read "IDD Brd(uA)"() -> (w591:string)
              n179 = call "Delay.vi"("milliseconds to wait"=u32 100, "error in (no error)"=w597) -> ("error out"=w595:errorcluster)  [unwired: 9 in]
              n180 = call "Ke2000 Single Reading.vi"("error in (no error)"=w595, "VISA resource name"=w586) -> ("error out"=w593:errorcluster, "VISA resource name out"=w578:refnum<visa-resource-name>, "uA"=w592:string)  [unwired: 5 in, 2 out]
              n181 = call "Substration.vi"("error in (no error)"=w593, "Input2"=w591, "Input1"=w592) -> ("error out"=w583:errorcluster, "In1 - In2"=w582:string)  [unwired: 7 in]
              "IDD_HD/CYC (uA)" <- w582
              n182 = for {
                N: 36 -> [_]
                shift-right: [w602] -> w579
                shift-left: w583 -> [w602]
                tunnel: w582 -> [w601]
                tunnel: [w601] -> w571 mode=indexing
                tunnel: w581 -> [w600]
                tunnel: [w600] -> w573 mode=indexing
              }
              n183 = flat-sequence {
                tunnel: w579 -> [w611]
                tunnel: [w608] -> w584
                tunnel: w574 -> [w607]
                tunnel: w573 -> [w606]
                tunnel: w572 -> [w605]
                tunnel: w571 -> [w604]
                tunnel: [w603] -> w570
                frame #0 {
                  n184 = Build Array (concatenate)(w607, w606, w605, w604) -> (w603:string[])
                  n185 = Select(t=WS105x_Run_Sequences."Save Data" ("WS105x Run Sequences"), s=w611, f=WS105x_Run_Sequences."Idd" ("WS105x Run Sequences")) -> (s? t:f=w608:T4)
                }
              }
            }
            frame "Idd" {
              n186 = call "Delay.vi"("milliseconds to wait"=u32 50, "error in (no error)"=w686) -> ("error out"=w688:errorcluster)  [unwired: 9 in]
              n187 = for {
                tunnel: [w714] -> w678
                tunnel: w687 -> [w713]
                tunnel: w688 -> [w709]
                tunnel: string[] ["0702013B3B3B", "070201000000"] -> [w705] mode=indexing
                tunnel: [w704] -> w679 mode=indexing
                tunnel: [w702] -> w684
                n188 = call "WSVCAP SHL Host TL RFFE Write - Multiple DUTs - Common Data.vi"("Data Out"=w705, "error in"=w709, "Log (T)"=FALSE) -> ("error out"=w710:errorcluster)  [unwired: 12 in]
                n189 = call "Delay.vi"("milliseconds to wait"=u32 100, "error in (no error)"=w710) -> ("error out"=w711:errorcluster)  [unwired: 9 in]
                n190 = call "Ke2000 Single Reading.vi"("error in (no error)"=w711, "VISA resource name"=w713) -> ("error out"=w708:errorcluster, "VISA resource name out"=w702:refnum<visa-resource-name>, "uA"=w707:string)  [unwired: 5 in, 2 out]
                n191 = local read "IDD Brd(uA)"() -> (w706:string)
                n192 = call "Substration.vi"("error in (no error)"=w708, "Input2"=w706, "Input1"=w707) -> ("error out"=w714:errorcluster, "In1 - In2"=w704:string)  [unwired: 7 in]
              }
              n193 = Index Array(array=w679, index=0) -> (element=w675:string)
              "NOM IDD OFF(uA)" <- w675
              n194 = Index Array(array=w679, index=0) -> (element=w676:string)
              "NOM IDD ON (uA)" <- w676
              n195 = for {
                N: 36 -> [_]
                shift-right: [w693] -> w677
                shift-left: w678 -> [w693]
                tunnel: w676 -> [w692]
                tunnel: [w692] -> w671 mode=indexing
                tunnel: w675 -> [w691]
                tunnel: [w691] -> w670 mode=indexing
              }
              n196 = flat-sequence {
                tunnel: w677 -> [w701]
                tunnel: [w698] -> w685
                tunnel: w672 -> [w697]
                tunnel: w671 -> [w696]
                tunnel: w670 -> [w695]
                tunnel: [w694] -> w669
                frame #0 {
                  n197 = Build Array (concatenate)(w697, w696, w695) -> (w694:string[])
                  n198 = Select(t=WS105x_Run_Sequences."Save Data" ("WS105x Run Sequences"), s=w701, f=WS105x_Run_Sequences."Stress" ("WS105x Run Sequences")) -> (s? t:f=w698:T4)
                }
              }
            }
            frame "Stress" {
              n199 = case shown="True" w739 {
                tunnel: [w781 w886] -> w721
                tunnel: [w782 w871] -> w730
                tunnel: [w780 w887] -> w728
                tunnel: w744 -> [w776 w875]
                tunnel: w735 -> [_ w877]
                tunnel: w743 -> [w774 w872]
                tunnel: [w778 w873] -> w724
                tunnel: w741 -> [w766 w869]
                tunnel: ["% Duty Cycle" "100" ("Data Out")] -> w726
                tunnel: "Real No. From\nLookup Table" -> [w764 w864]
                tunnel: w736 -> [w761 _]
                tunnel: w737 -> [w760 _]
                tunnel: w742 -> [w759 _]
                tunnel: w740 -> [w758 _]
                frame False {
                  # "Cycles in 1s"
                  # "Cycling"
                  n200 = case shown="True" w764 {
                    tunnel: w776 -> [w788 w794]
                    tunnel: w774 -> [w787 w793]
                    tunnel: [w786 w794] -> w773
                    tunnel: w766 -> [w785 _]
                    tunnel: [w784 w793] -> w772
                    tunnel: [u64 1000 ("y") u64 1 ("y")] -> w767
                    frame False {
                      n201 = case shown="8, Default" w785 {
                        tunnel: w787 -> [w790 _]
                        tunnel: [w790 "Cycle RP"] -> w784
                        tunnel: [w789 w791] -> w786
                        tunnel: w788 -> [w789 w791]
                        frame 0..7 {
                        }
                        frame 8, Default {
                        }
                      }
                    }
                    frame True {
                      # "Read real number\nfrom lookup table"
                    }
                  }
                  n202 = call "WSVCAP SHL Host TL RFFE Configure.vi"("RFFE Slave Address"=w758, "Clock Rate (Hz)"="SPI Clock Rate (Hz)", "error in"=w773) -> ("Actual Rate (Hz)"=→"AR Cycling(Hz)":dbl, "error out"=w763:errorcluster)  [unwired: 11 in]
                  n203 = Array Max & Min(array=w760) -> (max value=w770:dbl)  [unwired: 3 out]
                  n204 = Divide(x=1.0, y=w770) -> (x/y=w769:dbl)
                  n205 = To Unsigned Quad Integer(1:w769) -> (0:w768:u64)
                  n206 = Not(x=w759) -> (.not. x?=w765:bool)
                  n207 = case shown="False" w765 {
                    tunnel: [w797 w819] -> w782
                    tunnel: [w800 w818] -> w781
                    tunnel: [u64 1 w817] -> w780
                    tunnel: w763 -> [w798 w816]
                    tunnel: w772 -> [_ w815]
                    tunnel: w760 -> [_ w813]
                    tunnel: w768 -> [_ w812]
                    tunnel: w767 -> [_ w811]
                    tunnel: w766 -> [w796 _]
                    tunnel: w761 -> [_ w810]
                    frame False {
                      n208 = case shown="1, Default" w796 {
                        tunnel: w798 -> [w801 w803]
                        tunnel: [w801 w802] -> w797
                        frame 0 {
                        }
                        frame 1, Default {
                          n209 = flat-sequence {
                            tunnel: "Repeat Meas(s)" -> [w809]
                            tunnel: w803 -> [w806]
                            tunnel: [w806] -> w802
                            frame #0 {
                              n210 = Multiply(x=w809, y=u32 1000) -> (x*y=w808:u32)
                              n211 = Wait (ms)(milliseconds to wait=w808) -> ()  [unwired: 1 out]
                              n212 = local write "STATUS"("Verify Sockets waiting times..." ("STATUS")) -> ()
                            }
                          }
                        }
                      }
                      n213 = local read "stop During HD/Cycles"() -> (w800:bool)
                    }
                    frame True {
                      n214 = while {
                        tunnel: w815 -> [w839]
                        tunnel: [w826] -> w819
                        tunnel: [w831] -> w818
                        tunnel: w816 -> [w837]
                        tunnel: [w825] -> w817
                        tunnel: w810 -> [w836]
                        tunnel: w813 -> [w835]
                        tunnel: w812 -> [w822]
                        tunnel: w811 -> [w820]
                        i -> [w834]
                        stop <- w830 stop-if-true
                        # "At least 1 second before target"
                        # "Remaining Cycles"
                        # "Target Cycles"
                        # "Cycles in 1s"
                        n215 = To Unsigned Quad Integer(1:w839) -> (0:w838:u64)
                        n216 = case shown="0" w834 {
                          tunnel: [w847 w849] -> w828
                          tunnel: w837 -> [w848 w849]
                          tunnel: w836 -> [w846 _]
                          tunnel: w835 -> [w845 _]
                          frame 0 {
                            n217 = call "WSVCAP SHL Host TL RFFE Write Cycle - Multiple DUTs - Common Data.vi"("Data Out (Cycle Commands)"=w846, "Post Command Delay"=w845, "error in"=w848, "Log (T)"=FALSE) -> ("error out"=w847:errorcluster)  [unwired: 11 in]
                          }
                          frame 1, Default {
                          }
                        }
                        n218 = Multiply(x=w838, y=w820) -> (x*y=w825:u64)
                        n219 = call "WSVCAP SHL Host TL SPI_RFFE Query Cycle Count.vi"("error in"=w828) -> ("Cycle Count"=w824:u64, "error out"=w833:errorcluster)  [unwired: 13 in]
                        "Cycle Count" <- w824
                        n220 = Subtract(x=w825, y=w824) -> (x-y=w823:u64)
                        n221 = Greater Or Equal?(x=w824, y=w825) -> (x >= y?=w832:bool)
                        n222 = local read "stop During HD/Cycles"() -> (w831:bool)
                        n223 = Greater?(x=w823, y=w822) -> (0:w821:bool)
                        n224 = case shown="True" w832 {
                          tunnel: [w851 w854] -> w827
                          tunnel: w833 -> [w851 w853]
                          tunnel: [FALSE TRUE] -> w829
                          frame False {
                          }
                          frame True {
                            n225 = call "WSVCAP SHL Host TL SPI Stop Write Cycle.vi"("error in"=w853) -> ("error out"=w854:errorcluster)  [unwired: 14 in]
                          }
                        }
                        n226 = Or(x=w829, y=w831) -> (x .or. y?=w830:bool)
                        n227 = case shown="True" w821 {
                          tunnel: w827 -> [w840 w843]
                          tunnel: [w840 w842] -> w826
                          frame False {
                          }
                          frame True {
                            n228 = call "MISC Wait with Data Flow.vi"("Error In (no error)"=w843, "Wait Time (500ms)"=u32 50) -> ("Error Out"=w842:errorcluster)  [unwired: 7 in, 2 out]
                          }
                        }
                      }
                      n229 = local write "STATUS"("Parts are Cycling...." ("STATUS")) -> ()
                    }
                  }
                  n230 = local read "HD/CYC Temp"() -> (w777:i32)
                  n231 = Number To Engineering String(4:w777) -> (0:w778:string)  [unwired: 3 in]
                }
                frame True {
                  # "Hold Down"
                  n232 = case shown="False" w864 {
                    tunnel: w877 -> [w904 _]
                    tunnel: [w903 w916] -> w876
                    tunnel: w875 -> [w902 w917]
                    tunnel: [w901 w917] -> w874
                    tunnel: w872 -> [w900 w916]
                    tunnel: w869 -> [w899 _]
                    frame False {
                      n233 = case shown="1, Default" w904 {
                        tunnel: [w907 w914] -> w903
                        tunnel: w902 -> [w909 w915]
                        tunnel: [w908 w915] -> w901
                        tunnel: w900 -> [w906 _]
                        tunnel: w899 -> [w905 _]
                        frame 0 {
                          n234 = case shown="15, Default" w905 {
                            tunnel: [w910 "HD RP"] -> w907
                            tunnel: w909 -> [w911 w912]
                            tunnel: [w911 w912] -> w908
                            tunnel: w906 -> [w910 _]
                            frame 0..14 {
                            }
                            frame 15, Default {
                            }
                          }
                        }
                        frame 1, Default {
                          n235 = local read "HD RP"() -> (w914:dbl)
                        }
                      }
                    }
                    frame True {
                    }
                  }
                  n236 = call "WSVCAP SHL Host TL RFFE Write - Multiple DUTs - Common Data.vi"("Data Out"="Cmd To HD", "error in"=w874, "Log (T)"=FALSE) -> ("error out"=w860:errorcluster)  [unwired: 12 in]
                  n237 = call "Delay.vi"("milliseconds to wait"=u32 50, "error in (no error)"=w860) -> ("error out"=w857:errorcluster)  [unwired: 9 in]
                  n238 = for {
                    tunnel: string[] ["0761", "0762", "0763"] -> [w898] mode=indexing
                    tunnel: [w894] -> w856 mode=indexing
                    shift-right: [w891] -> w882
                    shift-left: w857 -> [w897]
                    i -> [w896]
                    n239 = call "WSVCAP SHL Host TL RFFE Read - Multiple DUTs - Common Data.vi"("Data Out"=w898, "error in"=w897, "Log (T)"=FALSE) -> ("RFFE Data In"=w893:string[], "error out"=w890:errorcluster)  [unwired: 11 in]
                    n240 = Index Array(array=w893, index=w896) -> (element=w892:string)
                    n241 = call "Delay.vi"("milliseconds to wait"=u32 10, "error in (no error)"=w890) -> ("error out"=w891:errorcluster)  [unwired: 9 in]
                    n242 = String Subset(string=w892, offset (0)=0) -> (substring=w894:string)  [unwired: 1 in]
                  }
                  "RB Reg for HD" <- w856
                  n243 = local read "No of HD/Cycle\nCompleted"() -> (w878:u64)
                  n244 = Greater?(x="HD_DC (Min)", y=w878) -> (0:w879:bool)
                  n245 = case shown="True" w879 {
                    tunnel: [_ w928] -> w884
                    tunnel: [w919 w927] -> w883
                    tunnel: w882 -> [w919 w926]
                    tunnel: w876 -> [w918 w925]
                    tunnel: [w918 w925] -> w881
                    frame False {
                    }
                    frame True {
                      n246 = Multiply(x=1000.0, y=w925) -> (x*y=w923:dbl)
                      n247 = Multiply(x=60.0, y=w923) -> (x*y=w921:dbl)
                      n248 = event shown="[0] Timeout" {
                        selector: _ -> [_ _]
                        dyn-events: _ -> [_ _]
                        timeout: w921 -> [_ _]
                        tunnel: ["stop During HD/Cycles" TRUE ("stop During HD/Cycles")] -> w928
                        tunnel: w926 -> [w929 w931]
                        tunnel: [w929 w931] -> w927
                        event Timeout {
                          n249 = event-data() -> ()  [unwired: 1 in, 2 out]
                        }
                        event "stop During HD/Cycles": Value Change {
                          n250 = event-data() -> ()  [unwired: 1 in, 2 out]
                        }
                      }
                      n251 = local write "STATUS"("Parts are Holding Down..." ("STATUS")) -> ()
                    }
                  }
                  n252 = Greater Or Equal?(x=w878, y="HD_DC (Min)") -> (x >= y?=w885:bool)
                  n253 = To Unsigned Quad Integer(1:w876) -> (0:w887:u64)
                  n254 = Add(x="Time All OFF (s)", y="Time All ON (s)") -> (x+y=w866:u32)
                  n255 = To Double Precision Float(number=w866) -> (double precision float=w865:dbl)
                  n256 = Divide(x=w865, y=60.0) -> (x/y=w867:dbl)
                  n257 = case shown="False" w885 {
                    tunnel: [w935 w951] -> w886
                    tunnel: [w936 w943] -> w871
                    tunnel: w883 -> [w936 w950]
                    tunnel: w884 -> [w935 w949]
                    tunnel: w881 -> [_ w948]
                    tunnel: [w934 w946] -> w873
                    tunnel: w867 -> [_ w940]
                    tunnel: "Time All OFF (s)" -> [_ w938]
                    tunnel: "Time All ON (s)" -> [_ w937]
                    frame False {
                      n258 = Number To Engineering String(4:"HD/CYC Temp") -> (0:w934:string)  [unwired: 3 in]
                    }
                    frame True {
                      n259 = Divide(x=w948, y=w940) -> (x/y=w947:dbl)
                      n260 = call "WSVCAP SHL Host TL RFFE Write - Multiple DUTs - Common Data.vi"("Data Out"="070201000000", "error in"=w950, "Log (T)"=FALSE) -> ("error out"=w953:errorcluster)  [unwired: 12 in]
                      n261 = Round To Nearest(number=w947) -> (nearest integer value=w942:dbl)
                      n262 = call "Delay.vi"("milliseconds to wait"=u32 50, "error in (no error)"=w953) -> ("error out"=w944:errorcluster)  [unwired: 9 in]
                      n263 = To Long Integer(number=w942) -> (32bit integer=w941:i32)
                      "No LPs to RP" <- w941
                      n264 = for {
                        N: w941 -> [_]
                        tunnel: w949 -> [w970]
                        tunnel: [w969] -> w951
                        tunnel: w944 -> [w961]
                        tunnel: [w960] -> w943
                        tunnel: w938 -> [w958]
                        tunnel: w937 -> [w957]
                        i -> [w968]
                        stop <- w969 stop-if-true
                        w959 = FALSE ("Log (T)")
                        n265 = local read "CP to HD/Cycle"() -> (w963:i32)
                        n266 = Increment(x=w968) -> (x+1=→"LPs Count":i32)
                        n267 = call "WSVCAP SHL Host TL RFFE Write - Multiple DUTs - Common Data.vi"("Data Out"="074776", "error in"=w961, "Log (T)"=w959) -> ("error out"=w956:errorcluster)  [unwired: 12 in]
                        n268 = call "WSVCAP SHL Host TL RFFE Write - Multiple DUTs - Common Data.vi"("Data Out"="0702013B3B3B", "error in"=w956, "Log (T)"=w959) -> ("error out"=w955:errorcluster)  [unwired: 12 in]
                        n269 = Index Array(array=string[] ["07476F", "074776", "074765", "074769", "07477B"], index=w963) -> (element=w966:string)
                        n270 = call "WSVCAP SHL Host TL RFFE Write - Multiple DUTs - Common Data.vi"("Data Out"=w966, "error in"=w955, "Log (T)"=w959) -> ("error out"=w965:errorcluster)  [unwired: 12 in]
                        n271 = flat-sequence {
                          tunnel: [w986] -> w964
                          tunnel: w965 -> [w983]
                          tunnel: w957 -> [w982]
                          frame #0 {
                            n272 = local write "STATUS"("Now HD ON Time..." ("STATUS")) -> ()
                            n273 = Multiply(x=w982, y=u32 1000) -> (x*y=w985:u32)
                            n274 = call "Delay.vi"("milliseconds to wait"=w985, "error in (no error)"=w983) -> ("error out"=w986:errorcluster)  [unwired: 9 in]
                          }
                        }
                        n275 = call "WSVCAP SHL Host TL RFFE Write - Multiple DUTs - Common Data.vi"("Data Out"="070201000000", "error in"=w964) -> ("error out"=w972:errorcluster)  [unwired: 13 in]
                        n276 = flat-sequence {
                          tunnel: w972 -> [w981]
                          tunnel: [w979] -> w960
                          tunnel: w958 -> [w976]
                          frame #0 {
                            n277 = local write "STATUS"("Now HD OFF Time..." ("STATUS")) -> ()
                            n278 = Multiply(x=w976, y=u32 1000) -> (x*y=w978:u32)
                            n279 = call "Delay.vi"("milliseconds to wait"=w978, "error in (no error)"=w981) -> ("error out"=w979:errorcluster)  [unwired: 9 in]
                          }
                        }
                        n280 = Unbundle By Name(w960) -> ("status"=w971:bool)
                        n281 = Or(x=w971, y=w970) -> (x .or. y?=w969:bool)
                      }
                      n282 = Number To Engineering String(4:"DC_Temp") -> (0:w946:string)  [unwired: 3 in]
                    }
                  }
                }
              }
              n283 = Add(x=w723, y=w728) -> (x+y=w722:u64)
              "No of HD/Cycle\nCompleted" <- w722
              n284 = Number To Engineering String(4:w722) -> (0:w727:string)  [unwired: 3 in]
              n285 = for {
                N: 36 -> [_]
                tunnel: [w748] -> w729
                tunnel: w730 -> [w748]
                tunnel: w727 -> [w747]
                tunnel: [w747] -> w717 mode=indexing
                tunnel: w726 -> [w746]
                tunnel: [w746] -> w719 mode=indexing
                tunnel: w724 -> [w745]
                tunnel: [w745] -> w718 mode=indexing
              }
              n286 = flat-sequence {
                tunnel: [w757] -> w734
                tunnel: w730 -> [w755]
                tunnel: w720 -> [w753]
                tunnel: w719 -> [w752]
                tunnel: w718 -> [w751]
                tunnel: w717 -> [w750]
                tunnel: [w749] -> w716
                frame #0 {
                  n287 = Build Array (concatenate)(w753, w752, w751, w750) -> (w749:string[])
                  n288 = Select(t=WS105x_Run_Sequences."Save Data" ("WS105x Run Sequences"), s=w755, f=WS105x_Run_Sequences."Meas CAP" ("WS105x Run Sequences")) -> (s? t:f=w757:T4)
                }
              }
            }
            frame "Meas CAP" {
              n289 = local read "Clock Rate (Hz)"() -> (w992:dbl)
              n290 = call "WSVCAP SHL Host TL RFFE Configure.vi"("RFFE Slave Address"=w991, "Clock Rate (Hz)"=w992, "error in"=w990) -> ("Actual Rate (Hz)"=w993:dbl, "error out"=w989:errorcluster)  [unwired: 11 in]
              n291 = local write "AR  Measurent(Hz)"(w993) -> ()
              n292 = stacked-sequence {
                seq-local: [w1065 _ _] -> [_ w1181 _]
                seq-local: [_ w1179 _] -> [_ _ w1263]
                tunnel: w989 -> [w1068 _ _]
                tunnel: w1032 -> [w1066 w1180 w1264]
                tunnel: w1031 -> [w1069 _ _]
                tunnel: w1030 -> [_ w1182 _]
                tunnel: w1029 -> [_ _ w1262]
                tunnel: w1028 -> [w1067 _ _]
                tunnel: [w1064 _ _] -> w1009
                tunnel: [_ w1177 _] -> w1017
                tunnel: w1016 -> [_ w1178 _]
                tunnel: w1015 -> [_ _ w1261]
                tunnel: [_ _ w1259] -> w1014
                tunnel: [_ _ w1260] -> w1013
                tunnel: [_ _ w1258] -> w1003
                tunnel: [w1063 _ _] -> w1005
                tunnel: [_ w1176 _] -> w1004
                tunnel: w996 -> [w1062 w1175 w1257]
                frame #0 {
                  n293 = case shown="True" w1062 {
                    tunnel: w1067 -> [w1078 _]
                    tunnel: w1069 -> [w1073 _]
                    tunnel: w1068 -> [w1077 w1174]
                    tunnel: [w1076 w1174] -> w1065
                    tunnel: [w1074 string[][] []] -> w1064
                    tunnel: w1066 -> [w1075 _]
                    tunnel: [w1070 string[] []] -> w1063
                    frame False {
                      n294 = Array Size(array=w1073) -> (size(s)=w1072:i32)
                      n295 = case shown="1" w1075 {
                        tunnel: w1072 -> [w1086 w1117 w1143]
                        tunnel: w1078 -> [w1085 w1116 w1148]
                        tunnel: w1073 -> [w1084 w1115 w1147]
                        tunnel: w1077 -> [w1083 w1114 w1146]
                        tunnel: [w1082 w1113 w1145] -> w1076
                        tunnel: [w1081 w1112 w1144] -> w1074
                        tunnel: string[] [] -> [w1080 w1111 w1142]
                        tunnel: [w1079 w1110 w1141] -> w1070
                        frame 0, Default {
                          n296 = for {
                            N: w1086 -> [_]
                            tunnel: w1085 -> [w1105]
                            tunnel: [w1089] -> w1081 mode=indexing
                            tunnel: w1084 -> [w1103]
                            tunnel: w1083 -> [w1094]
                            tunnel: [w1095] -> w1082
                            shift-right: [w1088] -> w1079
                            shift-left: w1080 -> [w1087]
                            i -> [w1090]
                            stop <- w1092 stop-if-true
                            n297 = Index Array(array=w1103, index=w1090) -> (element=w1102:string)
                            n298 = Index Array(array=w1105, index=w1090) -> (element=w1104:string)
                            n299 = local write "STATUS"(w1102) -> ()
                            n300 = call "WSVCAP SHL Host TL RFFE Write - Multiple DUTs - Common Data.vi"("Data Out"=w1104, "error in"=w1094, "Log (T)"=FALSE) -> ("error out"=w1097:errorcluster)  [unwired: 12 in]
                            n301 = call "Delay.vi"("milliseconds to wait"=u32 10, "error in (no error)"=w1097) -> ("error out"=w1101:errorcluster)  [unwired: 9 in]
                            n302 = call "WS1050 AD7747 READ 36 DUT.vi"("error in"=w1101, "Log (T)"=FALSE, "DUT Mask Mode (All)"=WSVCAP_SHL_I2C_DUT_Mask_Mode_Enum."C1") -> ("error out"=w1099:errorcluster, "AD7747 Values"=w1100:string[][])  [unwired: 7 in]
                            n303 = for {
                              tunnel: w1100 -> [w1108] mode=indexing
                              tunnel: w1099 -> [w1109]
                              tunnel: [w1109] -> w1095
                              tunnel: [w1106] -> w1089 mode=indexing
                              n304 = Index Array(array=w1108, index=1) -> (element=w1106:string)
                            }
                            n305 = Build Array (concatenate)(w1087, w1089) -> (w1088:string[])
                            n306 = Unbundle By Name(w1095) -> ("status"=w1092:bool)
                          }
                        }
                        frame 1 {
                          n307 = for {
                            N: w1117 -> [_]
                            tunnel: w1116 -> [w1136]
                            tunnel: [w1120] -> w1112 mode=indexing
                            tunnel: w1115 -> [w1134]
                            tunnel: w1114 -> [w1125]
                            tunnel: [w1126] -> w1113
                            shift-right: [w1119] -> w1110
                            shift-left: w1111 -> [w1118]
                            i -> [w1121]
                            stop <- w1123 stop-if-true
                            n308 = Index Array(array=w1134, index=w1121) -> (element=w1133:string)
                            n309 = Index Array(array=w1136, index=w1121) -> (element=w1135:string)
                            n310 = local write "STATUS"(w1133) -> ()
                            n311 = call "WSVCAP SHL Host TL RFFE Write - Multiple DUTs - Common Data.vi"("Data Out"=w1135, "error in"=w1125, "Log (T)"=FALSE) -> ("error out"=w1128:errorcluster)  [unwired: 12 in]
                            n312 = call "Delay.vi"("milliseconds to wait"=u32 10, "error in (no error)"=w1128) -> ("error out"=w1132:errorcluster)  [unwired: 9 in]
                            n313 = call "WS1050 AD7747 READ 36 DUT.vi"("error in"=w1132, "Log (T)"=FALSE, "DUT Mask Mode (All)"=WSVCAP_SHL_I2C_DUT_Mask_Mode_Enum."C2") -> ("error out"=w1130:errorcluster, "AD7747 Values"=w1131:string[][])  [unwired: 7 in]
                            n314 = for {
                              tunnel: w1131 -> [w1139] mode=indexing
                              tunnel: w1130 -> [w1140]
                              tunnel: [w1140] -> w1126
                              tunnel: [w1137] -> w1120 mode=indexing
                              n315 = Index Array(array=w1139, index=3) -> (element=w1137:string)
                            }
                            n316 = Build Array (concatenate)(w1118, w1120) -> (w1119:string[])
                            n317 = Unbundle By Name(w1126) -> ("status"=w1123:bool)
                          }
                        }
                        frame 2 {
                          n318 = for {
                            N: w1143 -> [_]
                            tunnel: w1148 -> [w1167]
                            tunnel: [w1151] -> w1144 mode=indexing
                            tunnel: w1147 -> [w1165]
                            tunnel: w1146 -> [w1156]
                            tunnel: [w1157] -> w1145
                            shift-right: [w1150] -> w1141
                            shift-left: w1142 -> [w1149]
                            i -> [w1152]
                            stop <- w1154 stop-if-true
                            n319 = Index Array(array=w1167, index=w1152) -> (element=w1166:string)
                            n320 = Index Array(array=w1165, index=w1152) -> (element=w1164:string)
                            n321 = local write "STATUS"(w1164) -> ()
                            n322 = call "WSVCAP SHL Host TL RFFE Write - Multiple DUTs - Common Data.vi"("Data Out"=w1166, "error in"=w1156, "Log (T)"=FALSE) -> ("error out"=w1159:errorcluster)  [unwired: 12 in]
                            n323 = call "Delay.vi"("milliseconds to wait"=u32 10, "error in (no error)"=w1159) -> ("error out"=w1163:errorcluster)  [unwired: 9 in]
                            n324 = call "WS1050 AD7747 READ 36 DUT.vi"("error in"=w1163, "Log (T)"=FALSE, "DUT Mask Mode (All)"=WSVCAP_SHL_I2C_DUT_Mask_Mode_Enum."C3") -> ("error out"=w1161:errorcluster, "AD7747 Values"=w1162:string[][])  [unwired: 7 in]
                            n325 = for {
                              tunnel: w1162 -> [w1170] mode=indexing
                              tunnel: w1161 -> [w1171]
                              tunnel: [w1171] -> w1157
                              tunnel: [w1168] -> w1151 mode=indexing
                              n326 = Index Array(array=w1170, index=5) -> (element=w1168:string)
                            }
                            n327 = Build Array (concatenate)(w1149, w1151) -> (w1150:string[])
                            n328 = Unbundle By Name(w1157) -> ("status"=w1154:bool)
                          }
                        }
                      }
                    }
                    frame True {
                    }
                  }
                  "CAP_C1" <- w1064
                }
                frame #1 {
                  n329 = case shown="False" w1175 {
                    tunnel: w1182 -> [w1186 _]
                    tunnel: w1178 -> [w1191 _]
                    tunnel: [w1190 w1256] -> w1179
                    tunnel: w1181 -> [w1189 w1256]
                    tunnel: [w1188 string[][] []] -> w1177
                    tunnel: w1180 -> [w1187 _]
                    tunnel: [w1184 string[] []] -> w1176
                    frame False {
                      n330 = Array Size(array=w1186) -> (size(s)=w1185:i32)
                      n331 = case shown="1" w1187 {
                        tunnel: w1185 -> [w1199 w1230]
                        tunnel: w1186 -> [w1198 w1229]
                        tunnel: w1191 -> [w1197 w1228]
                        tunnel: [w1196 w1227] -> w1190
                        tunnel: w1189 -> [w1195 w1226]
                        tunnel: [w1194 w1225] -> w1188
                        tunnel: [w1193 w1223] -> w1184
                        tunnel: string[] [] -> [w1192 w1224]
                        frame 0, 2, Default {
                          n332 = for {
                            N: w1199 -> [_]
                            tunnel: w1197 -> [w1218]
                            tunnel: [w1202] -> w1194 mode=indexing
                            tunnel: w1198 -> [w1216]
                            tunnel: w1195 -> [w1207]
                            tunnel: [w1208] -> w1196
                            shift-right: [w1201] -> w1193
                            shift-left: w1192 -> [w1200]
                            i -> [w1203]
                            stop <- w1205 stop-if-true
                            n333 = Index Array(array=w1218, index=w1203) -> (element=w1217:string)
                            n334 = Index Array(array=w1216, index=w1203) -> (element=w1215:string)
                            n335 = local write "STATUS"(w1215) -> ()
                            n336 = call "WSVCAP SHL Host TL RFFE Write - Multiple DUTs - Common Data.vi"("Data Out"=w1217, "error in"=w1207, "Log (T)"=FALSE) -> ("error out"=w1210:errorcluster)  [unwired: 12 in]
                            n337 = call "Delay.vi"("milliseconds to wait"=u32 10, "error in (no error)"=w1210) -> ("error out"=w1214:errorcluster)  [unwired: 9 in]
                            n338 = call "WS1050 AD7747 READ 36 DUT.vi"("error in"=w1214, "Log (T)"=FALSE, "DUT Mask Mode (All)"=WSVCAP_SHL_I2C_DUT_Mask_Mode_Enum."C2") -> ("error out"=w1212:errorcluster, "AD7747 Values"=w1213:string[][])  [unwired: 7 in]
                            n339 = for {
                              tunnel: w1213 -> [w1221] mode=indexing
                              tunnel: w1212 -> [w1222]
                              tunnel: [w1222] -> w1208
                              tunnel: [w1219] -> w1202 mode=indexing
                              n340 = Index Array(array=w1221, index=3) -> (element=w1219:string)
                            }
                            n341 = Unbundle By Name(w1208) -> ("status"=w1205:bool)
                            n342 = Build Array (concatenate)(w1200, w1202) -> (w1201:string[])
                          }
                        }
                        frame 1 {
                          n343 = for {
                            N: w1230 -> [_]
                            tunnel: w1228 -> [w1249]
                            tunnel: [w1233] -> w1225 mode=indexing
                            tunnel: w1229 -> [w1247]
                            tunnel: w1226 -> [w1238]
                            tunnel: [w1239] -> w1227
                            shift-right: [w1232] -> w1223
                            shift-left: w1224 -> [w1231]
                            i -> [w1234]
                            stop <- w1236 stop-if-true
                            n344 = Index Array(array=w1247, index=w1234) -> (element=w1246:string)
                            n345 = Index Array(array=w1249, index=w1234) -> (element=w1248:string)
                            n346 = local write "STATUS"(w1246) -> ()
                            n347 = call "WSVCAP SHL Host TL RFFE Write - Multiple DUTs - Common Data.vi"("Data Out"=w1248, "error in"=w1238, "Log (T)"=FALSE) -> ("error out"=w1241:errorcluster)  [unwired: 12 in]
                            n348 = call "Delay.vi"("milliseconds to wait"=u32 10, "error in (no error)"=w1241) -> ("error out"=w1245:errorcluster)  [unwired: 9 in]
                            n349 = call "WS1050 AD7747 READ 36 DUT.vi"("error in"=w1245, "Log (T)"=FALSE, "DUT Mask Mode (All)"=WSVCAP_SHL_I2C_DUT_Mask_Mode_Enum."C1") -> ("error out"=w1243:errorcluster, "AD7747 Values"=w1244:string[][])  [unwired: 7 in]
                            n350 = for {
                              tunnel: w1244 -> [w1252] mode=indexing
                              tunnel: w1243 -> [w1253]
                              tunnel: [w1253] -> w1239
                              tunnel: [w1250] -> w1233 mode=indexing
                              n351 = Index Array(array=w1252, index=1) -> (element=w1250:string)
                            }
                            n352 = Unbundle By Name(w1239) -> ("status"=w1236:bool)
                            n353 = Build Array (concatenate)(w1231, w1233) -> (w1232:string[])
                          }
                        }
                      }
                    }
                    frame True {
                    }
                  }
                  "CAP_C2" <- w1177
                }
                frame #2 {
                  n354 = case shown="False" w1257 {
                    tunnel: w1262 -> [w1268 _]
                    tunnel: w1261 -> [w1273 _]
                    tunnel: w1263 -> [w1272 w1337]
                    tunnel: [w1271 string[][] []] -> w1259
                    tunnel: w1264 -> [w1270 _]
                    tunnel: [w1269 w1337] -> w1260
                    tunnel: [w1265 string[] []] -> w1258
                    frame False {
                      n355 = Array Size(array=w1268) -> (size(s)=w1267:i32)
                      n356 = case shown="2" w1270 {
                        tunnel: w1268 -> [w1281 w1312]
                        tunnel: w1273 -> [w1280 w1311]
                        tunnel: w1272 -> [w1279 w1310]
                        tunnel: [w1278 w1309] -> w1269
                        tunnel: [w1277 w1308] -> w1271
                        tunnel: w1267 -> [w1276 w1307]
                        tunnel: string[] [] -> [w1275 w1306]
                        tunnel: [w1274 w1305] -> w1265
                        frame 0, 1, Default {
                          n357 = for {
                            N: w1276 -> [_]
                            tunnel: w1280 -> [w1300]
                            tunnel: [w1284] -> w1277 mode=indexing
                            tunnel: w1281 -> [w1298]
                            tunnel: w1279 -> [w1289]
                            tunnel: [w1290] -> w1278
                            shift-right: [w1283] -> w1274
                            shift-left: w1275 -> [w1282]
                            i -> [w1285]
                            stop <- w1287 stop-if-true
                            n358 = Index Array(array=w1298, index=w1285) -> (element=w1297:string)
                            n359 = Index Array(array=w1300, index=w1285) -> (element=w1299:string)
                            n360 = local write "STATUS"(w1297) -> ()
                            n361 = call "WSVCAP SHL Host TL RFFE Write - Multiple DUTs - Common Data.vi"("Data Out"=w1299, "error in"=w1289, "Log (T)"=FALSE) -> ("error out"=w1292:errorcluster)  [unwired: 12 in]
                            n362 = call "Delay.vi"("milliseconds to wait"=u32 10, "error in (no error)"=w1292) -> ("error out"=w1296:errorcluster)  [unwired: 9 in]
                            n363 = call "WS1050 AD7747 READ 36 DUT.vi"("error in"=w1296, "Log (T)"=FALSE, "DUT Mask Mode (All)"=WSVCAP_SHL_I2C_DUT_Mask_Mode_Enum."C3") -> ("error out"=w1294:errorcluster, "AD7747 Values"=w1295:string[][])  [unwired: 7 in]
                            n364 = for {
                              tunnel: w1295 -> [w1303] mode=indexing
                              tunnel: w1294 -> [w1304]
                              tunnel: [w1304] -> w1290
                              tunnel: [w1301] -> w1284 mode=indexing
                              n365 = Index Array(array=w1303, index=5) -> (element=w1301:string)
                            }
                            n366 = Build Array (concatenate)(w1282, w1284) -> (w1283:string[])
                            n367 = Unbundle By Name(w1290) -> ("status"=w1287:bool)
                          }
                        }
                        frame 2 {
                          n368 = for {
                            N: w1307 -> [_]
                            tunnel: w1311 -> [w1330]
                            tunnel: [w1315] -> w1308 mode=indexing
                            tunnel: w1312 -> [w1328]
                            tunnel: w1310 -> [w1319]
                            tunnel: [w1320] -> w1309
                            shift-right: [w1314] -> w1305
                            shift-left: w1306 -> [w1313]
                            i -> [w1316]
                            stop <- w1317 stop-if-true
                            n369 = Index Array(array=w1328, index=w1316) -> (element=w1327:string)
                            n370 = Index Array(array=w1330, index=w1316) -> (element=w1329:string)
                            n371 = local write "STATUS"(w1327) -> ()
                            n372 = call "WSVCAP SHL Host TL RFFE Write - Multiple DUTs - Common Data.vi"("Data Out"=w1329, "error in"=w1319, "Log (T)"=FALSE) -> ("error out"=w1322:errorcluster)  [unwired: 12 in]
                            n373 = call "Delay.vi"("milliseconds to wait"=u32 10, "error in (no error)"=w1322) -> ("error out"=w1326:errorcluster)  [unwired: 9 in]
                            n374 = call "WS1050 AD7747 READ 36 DUT.vi"("error in"=w1326, "DUT Mask Mode (All)"=WSVCAP_SHL_I2C_DUT_Mask_Mode_Enum."C1") -> ("error out"=w1324:errorcluster, "AD7747 Values"=w1325:string[][])  [unwired: 8 in]
                            n375 = for {
                              tunnel: w1325 -> [w1333] mode=indexing
                              tunnel: w1324 -> [w1334]
                              tunnel: [w1334] -> w1320
                              tunnel: [w1331] -> w1315 mode=indexing
                              n376 = Index Array(array=w1333, index=1) -> (element=w1331:string)
                            }
                            n377 = Build Array (concatenate)(w1313, w1315) -> (w1314:string[])
                            n378 = Unbundle By Name(w1320) -> ("status"=w1317:bool)
                          }
                        }
                      }
                    }
                    frame True {
                    }
                  }
                  "CAP_C3" <- w1259
                }
              }
              n379 = call "WS1050 Delta C Calculation.vi"("error in (no error)"=w1013, "DCap Target(pF)"=w1008, "Input"=w1009) -> ("error out"=w1026:errorcluster, "Total Bank Delta C(pF)"=w1020:string[], "% Bank DeltaC"=w1023:string[])  [unwired: 3 in, 3 out]
              n380 = call "WS1050 Delta C Calculation.vi"("error in (no error)"=w1013, "DCap Target(pF)"=w1008, "Input"=w1017) -> ("error out"=w1027:errorcluster, "Total Bank Delta C(pF)"=w1019:string[], "% Bank DeltaC"=w1022:string[])  [unwired: 3 in, 3 out]
              n381 = call "WS1050 Delta C Calculation.vi"("error in (no error)"=w1013, "DCap Target(pF)"=w1008, "Input"=w1014) -> ("error out"=w1025:errorcluster, "Total Bank Delta C(pF)"=w1018:string[], "% Bank DeltaC"=w1021:string[])  [unwired: 3 in, 3 out]
              n382 = Merge Errors(w1026, w1027, w1025) -> (w1024:errorcluster)
              n383 = case shown="0" w994 {
                tunnel: w1024 -> [w1053 w1061]
                tunnel: [w1053 w1061] -> w998
                tunnel: w1023 -> [w1049 w1057]
                tunnel: w1022 -> [w1048 w1056]
                tunnel: w1021 -> [w1047 w1055]
                tunnel: w1020 -> [w1052 w1060]
                tunnel: [w1052 w1060] -> w1002
                tunnel: w1019 -> [w1051 w1059]
                tunnel: [w1051 w1059] -> w1001
                tunnel: w1018 -> [w1050 w1058]
                tunnel: [w1050 w1058] -> w1000
                frame 0 {
                  n384 = Build Array(w1049, w1048, w1047) -> (→"% Delta C_T0":string[][])
                }
                frame 1, Default {
                  n385 = Build Array(w1057, w1056, w1055) -> (→"% Delta C":string[][])
                }
              }
              "Total Delta C1(pF)" <- w1002
              "Total Delta C2(pF)" <- w1001
              "Total Delta C3(pF)" <- w1000
              n386 = flat-sequence {
                tunnel: [w1043] -> w1007
                tunnel: w998 -> [w1042]
                tunnel: w1006 -> [w1041]
                tunnel: w1005 -> [w1040]
                tunnel: [w1039] -> _
                tunnel: w1004 -> [w1039]
                tunnel: w1003 -> [w1038]
                tunnel: w1002 -> [w1037]
                tunnel: [w1036] -> _
                tunnel: w1001 -> [w1036]
                tunnel: [w1035] -> _
                tunnel: w1000 -> [w1035]
                tunnel: [w1034] -> w999
                tunnel: w998 -> [w1033]
                tunnel: [w1033] -> w997
                frame #0 {
                  n387 = Build Array (concatenate)(w1041, w1040, w1039, w1038, w1037, w1036, w1035) -> (w1034:string[])
                  n388 = Select(t=WS105x_Run_Sequences."Save Data" ("WS105x Run Sequences"), s=w1042, f=WS105x_Run_Sequences."VPI" ("WS105x Run Sequences")) -> (s? t:f=w1043:T4)
                }
              }
            }
            frame "VPI" {
              n389 = case shown="True" w1354 {
                tunnel: [w1377 w1391] -> w1345
                tunnel: w1357 -> [_ w1411]
                tunnel: w1356 -> [_ w1396]
                tunnel: w1355 -> [_ w1392]
                tunnel: w1360 -> [w1380 w1410]
                tunnel: w1359 -> [_ w1397]
                tunnel: w1358 -> [_ w1393]
                tunnel: w1361 -> [w1378 w1407]
                tunnel: ["na" ("string") w1398] -> _
                tunnel: [w1374 w1395] -> w1352
                tunnel: [w1374 w1394] -> w1351
                tunnel: [w1374 w1390] -> w1350
                tunnel: [w1372 w1389] -> w1342
                tunnel: [w1372 w1388] -> w1341
                tunnel: [w1372 w1387] -> w1340
                frame False {
                  n390 = Array Size(array=w1380) -> (size(s)=w1379:i32)
                  n391 = for {
                    N: w1379 -> [_]
                    tunnel: [w1383] -> w1376 mode=indexing
                    tunnel: w1378 -> [w1384]
                    tunnel: [w1384] -> w1377
                    shift-right: [w1382] -> w1372
                    shift-left: string[] [] -> [w1381]
                    n392 = for {
                      N: 36 -> [_]
                      tunnel: [""] -> w1383 mode=indexing
                    }
                    n393 = Build Array (concatenate)(w1381, w1383) -> (w1382:string[])
                  }
                  n394 = Transpose 2D Array(2D array=w1376) -> (transposed array=w1374:string[][])
                }
                frame True {
                  w1408 = FALSE ("Log (T)")
                  # "Set CP VPI"
                  n395 = call "WSVCAP SHL Host TL RFFE Write - Multiple DUTs - Common Data.vi"("Data Out"="074820", "error in"=w1407, "Log (T)"=w1408) -> ("error out"=w1405:errorcluster)  [unwired: 12 in]
                  n396 = call "Delay.vi"("milliseconds to wait"=u32 10, "error in (no error)"=w1405) -> ("error out"=w1402:errorcluster)  [unwired: 9 in]
                  n397 = case shown="0, Default" "CP VPI" {
                    selector: "CP VPI" -> [w1508 w1513 w1518 w1523 w1528 w1533 w1538 w1543 w1547]
                    tunnel: string[] ["07476F", "074776", "074765", "074769", "07477B", "07477C", "07477D", "074779", "07476B"] -> [w1509 w1514 w1519 w1524 w1529 w1534 w1539 w1544 w1549]
                    tunnel: [w1507 w1512 w1517 w1522 w1527 w1532 w1537 w1542 w1548] -> w1401
                    tunnel: ["35.0" ("Data Out") "27.5" ("Data Out") "30.5" ("Data Out") "44.0" ("Data Out") "50.0" ("Data Out") "55.0" ("Data Out") "42.5" ("Data Out") "32.0" ("Data Out") "40.25" ("Data Out")] -> w1398
                    tunnel: [w1505 w1510 w1515 w1520 w1525 w1530 w1535 w1540 w1545] -> w1403
                    tunnel: w1402 -> [w1505 w1510 w1515 w1520 w1525 w1530 w1535 w1540 w1545]
                    frame 0, Default {
                      n398 = Index Array(array=w1509, index=w1508) -> (element=w1507:string)
                    }
                    frame 2 {
                      n399 = Index Array(array=w1514, index=w1513) -> (element=w1512:string)
                    }
                    frame 3 {
                      n400 = Index Array(array=w1519, index=w1518) -> (element=w1517:string)
                    }
                    frame 4 {
                      n401 = Index Array(array=w1524, index=w1523) -> (element=w1522:string)
                    }
                    frame 5 {
                      n402 = Index Array(array=w1529, index=w1528) -> (element=w1527:string)
                    }
                    frame 6 {
                      n403 = Index Array(array=w1534, index=w1533) -> (element=w1532:string)
                    }
                    frame 7 {
                      n404 = Index Array(array=w1539, index=w1538) -> (element=w1537:string)
                    }
                    frame 8 {
                      n405 = Index Array(array=w1544, index=w1543) -> (element=w1542:string)
                    }
                    frame 1 {
                      n406 = Index Array(array=w1549, index=w1547) -> (element=w1548:string)
                    }
                  }
                  n407 = call "WSVCAP SHL Host TL RFFE Write - Multiple DUTs - Common Data.vi"("Data Out"=w1401, "error in"=w1403, "Log (T)"=w1408) -> ("error out"=w1409:errorcluster)  [unwired: 12 in]
                  n408 = stacked-sequence {
                    seq-local: [w1415 _ _] -> [_ w1450 _]
                    seq-local: [_ w1445 _] -> [_ _ w1479]
                    tunnel: w1411 -> [w1418 _ _]
                    tunnel: w1410 -> [w1417 _ _]
                    tunnel: w1409 -> [w1416 _ _]
                    tunnel: w1397 -> [_ w1448 _]
                    tunnel: w1396 -> [_ w1447 _]
                    tunnel: [_ w1446 _] -> w1394
                    tunnel: [w1414 _ _] -> w1395
                    tunnel: w1393 -> [_ _ w1480]
                    tunnel: w1392 -> [_ _ w1478]
                    tunnel: [_ _ w1477] -> w1391
                    tunnel: [_ _ w1476] -> w1390
                    tunnel: [w1412 _ _] -> w1389
                    tunnel: [_ w1443 _] -> w1388
                    tunnel: [_ _ w1474] -> w1387
                    frame #0 {
                      n409 = Array Size(array=w1417) -> (size(s)=w1419:i32)
                      n410 = for {
                        N: w1419 -> [_]
                        tunnel: w1418 -> [w1438]
                        tunnel: [w1422] -> w1414 mode=indexing
                        tunnel: w1417 -> [w1436]
                        tunnel: w1416 -> [w1426]
                        tunnel: [w1423] -> w1415
                        shift-right: [w1421] -> w1412
                        shift-left: string[] [] -> [w1420]
                        i -> [w1435]
                        stop <- w1424 stop-if-true
                        n411 = Index Array(array=w1438, index=w1435) -> (element=w1437:string)
                        n412 = Index Array(array=w1436, index=w1435) -> (element=w1434:string)
                        n413 = local write "STATUS"(w1434) -> ()
                        n414 = call "WSVCAP SHL Host TL RFFE Write - Multiple DUTs - Common Data.vi"("Data Out"=w1437, "error in"=w1426, "Log (T)"=FALSE) -> ("error out"=w1433:errorcluster)  [unwired: 12 in]
                        n415 = call "Delay.vi"("milliseconds to wait"=u32 10, "error in (no error)"=w1433) -> ("error out"=w1429:errorcluster)  [unwired: 9 in]
                        n416 = call "WS1050 AD7747 READ 36 DUT.vi"("error in"=w1429, "Log (T)"=FALSE, "DUT Mask Mode (All)"=WSVCAP_SHL_I2C_DUT_Mask_Mode_Enum."C1") -> ("error out"=w1431:errorcluster, "AD7747 Values"=w1430:string[][])  [unwired: 7 in]
                        n417 = for {
                          tunnel: [w1441] -> w1422 mode=indexing
                          tunnel: w1431 -> [w1440]
                          tunnel: [w1440] -> w1423
                          tunnel: w1430 -> [w1439] mode=indexing
                          n418 = Index Array(array=w1439, index=1) -> (element=w1441:string)
                        }
                        n419 = Build Array (concatenate)(w1420, w1422) -> (w1421:string[])
                        n420 = Unbundle By Name(w1423) -> ("status"=w1424:bool)
                      }
                    }
                    frame #1 {
                      n421 = Array Size(array=w1448) -> (size(s)=w1449:i32)
                      n422 = for {
                        N: w1449 -> [_]
                        tunnel: w1447 -> [w1469]
                        tunnel: [w1453] -> w1446 mode=indexing
                        tunnel: w1448 -> [w1467]
                        tunnel: w1450 -> [w1456]
                        tunnel: [w1458] -> w1445
                        shift-right: [w1452] -> w1443
                        shift-left: string[] [] -> [w1451]
                        i -> [w1466]
                        stop <- w1454 stop-if-true
                        n423 = Index Array(array=w1469, index=w1466) -> (element=w1468:string)
                        n424 = Index Array(array=w1467, index=w1466) -> (element=w1465:string)
                        n425 = call "WSVCAP SHL Host TL RFFE Write - Multiple DUTs - Common Data.vi"("Data Out"=w1468, "error in"=w1456, "Log (T)"=FALSE) -> ("error out"=w1464:errorcluster)  [unwired: 12 in]
                        n426 = local write "STATUS"(w1465) -> ()
                        n427 = call "Delay.vi"("milliseconds to wait"=u32 10, "error in (no error)"=w1464) -> ("error out"=w1460:errorcluster)  [unwired: 9 in]
                        n428 = call "WS1050 AD7747 READ 36 DUT.vi"("error in"=w1460, "Log (T)"=FALSE, "DUT Mask Mode (All)"=WSVCAP_SHL_I2C_DUT_Mask_Mode_Enum."C2") -> ("error out"=w1462:errorcluster, "AD7747 Values"=w1461:string[][])  [unwired: 7 in]
                        n429 = for {
                          tunnel: [w1472] -> w1453 mode=indexing
                          tunnel: w1462 -> [w1471]
                          tunnel: [w1471] -> w1458
                          tunnel: w1461 -> [w1470] mode=indexing
                          n430 = Index Array(array=w1470, index=3) -> (element=w1472:string)
                        }
                        n431 = Build Array (concatenate)(w1451, w1453) -> (w1452:string[])
                        n432 = Unbundle By Name(w1458) -> ("status"=w1454:bool)
                      }
                    }
                    frame #2 {
                      n433 = Array Size(array=w1480) -> (size(s)=w1481:i32)
                      n434 = for {
                        N: w1481 -> [_]
                        tunnel: w1478 -> [w1500]
                        tunnel: [w1484] -> w1476 mode=indexing
                        tunnel: w1480 -> [w1498]
                        tunnel: w1479 -> [w1487]
                        tunnel: [w1489] -> w1477
                        shift-right: [w1483] -> w1474
                        shift-left: string[] [] -> [w1482]
                        i -> [w1497]
                        stop <- w1485 stop-if-true
                        n435 = Index Array(array=w1500, index=w1497) -> (element=w1499:string)
                        n436 = Index Array(array=w1498, index=w1497) -> (element=w1496:string)
                        n437 = call "WSVCAP SHL Host TL RFFE Write - Multiple DUTs - Common Data.vi"("Data Out"=w1499, "error in"=w1487, "Log (T)"=FALSE) -> ("error out"=w1495:errorcluster)  [unwired: 12 in]
                        n438 = local write "STATUS"(w1496) -> ()
                        n439 = call "Delay.vi"("milliseconds to wait"=u32 10, "error in (no error)"=w1495) -> ("error out"=w1491:errorcluster)  [unwired: 9 in]
                        n440 = call "WS1050 AD7747 READ 36 DUT.vi"("error in"=w1491, "Log (T)"=FALSE, "DUT Mask Mode (All)"=WSVCAP_SHL_I2C_DUT_Mask_Mode_Enum."C3") -> ("error out"=w1493:errorcluster, "AD7747 Values"=w1492:string[][])  [unwired: 7 in]
                        n441 = for {
                          tunnel: [w1503] -> w1484 mode=indexing
                          tunnel: w1493 -> [w1502]
                          tunnel: [w1502] -> w1489
                          tunnel: w1492 -> [w1501] mode=indexing
                          n442 = Index Array(array=w1501, index=5) -> (element=w1503:string)
                        }
                        n443 = Build Array (concatenate)(w1482, w1484) -> (w1483:string[])
                        n444 = Unbundle By Name(w1489) -> ("status"=w1485:bool)
                      }
                    }
                  }
                }
              }
              "VPI C1" <- w1352
              "VPI C2" <- w1351
              "VPI C3" <- w1350
              n445 = flat-sequence {
                tunnel: [w1369] -> w1346
                tunnel: w1345 -> [w1368]
                tunnel: [w1367] -> w1344
                tunnel: w1345 -> [w1367]
                tunnel: w1343 -> [w1366]
                tunnel: w1342 -> [w1365]
                tunnel: w1341 -> [w1364]
                tunnel: w1340 -> [w1363]
                tunnel: [w1362] -> w1339
                frame #0 {
                  n446 = Build Array (concatenate)(w1366, w1365, w1364, w1363) -> (w1362:string[])
                  n447 = Select(t=WS105x_Run_Sequences."Save Data" ("WS105x Run Sequences"), s=w1368, f=WS105x_Run_Sequences."VSA" ("WS105x Run Sequences")) -> (s? t:f=w1369:T4)
                }
              }
            }
            frame "VSA" {
              # "VSA Testing"
              n448 = case shown="False" w1557 {
                tunnel: w1570 -> [w1690 w1695]
                tunnel: [w1691 w1694] -> w1572
                frame False {
                  n449 = call "WSVCAP SHL Host TL RFFE Write - Multiple DUTs - Common Data.vi"("Data Out"="074820", "error in"=w1690, "Log (T)"=FALSE) -> ("error out"=w1691:errorcluster)  [unwired: 12 in]
                }
                frame True {
                  n450 = call "WSVCAP SHL Host TL RFFE Write - Multiple DUTs - Common Data.vi"("Data Out"="074800", "error in"=w1695, "Log (T)"=FALSE) -> ("error out"=w1694:errorcluster)  [unwired: 12 in]
                }
              }
              n451 = call "Delay.vi"("milliseconds to wait"=u32 10, "error in (no error)"=w1572) -> ("error out"=w1568:errorcluster)  [unwired: 9 in]
              n452 = case shown="True" w1563 {
                tunnel: w1568 -> [w1605 w1629]
                tunnel: [w1604 w1628] -> w1579
                tunnel: [w1609 w1635] -> w1588
                tunnel: w1569 -> [w1609 w1634]
                tunnel: [w1606 w1632] -> w1584
                tunnel: [w1606 w1631] -> w1581
                tunnel: [w1606 w1630] -> w1578
                tunnel: [w1607 w1633] -> w1585
                tunnel: "VSA Voltage(V)" -> [_ w1627]
                tunnel: [w1603 w1622] -> w1556
                tunnel: [w1601 w1623] -> w1554
                tunnel: [w1601 w1624] -> w1553
                tunnel: [w1601 w1625] -> w1552
                frame False {
                  w1602 = string[] []
                  n453 = for {
                    tunnel: dbl[] [0.0, 0.0, 0.0] -> [w1618] mode=indexing
                    tunnel: [w1615] -> w1607 mode=indexing
                    tunnel: [w1613] -> w1606 mode=indexing
                    tunnel: w1605 -> [w1616]
                    tunnel: [w1616] -> w1604
                    shift-right: [w1614] -> w1603
                    shift-left: w1602 -> [w1612]
                    shift-right: [w1610] -> w1601
                    shift-left: w1602 -> [w1611]
                    n454 = Number To Fractional String(number=w1618) -> (F-format string=w1619:string)  [unwired: 3 in]
                    n455 = for {
                      N: 36 -> [_]
                      tunnel: w1619 -> [w1621]
                      tunnel: [w1621] -> w1615 mode=indexing
                      tunnel: [""] -> w1613 mode=indexing
                    }
                    n456 = Build Array (concatenate)(w1612, w1615) -> (w1614:string[])
                    n457 = Build Array (concatenate)(w1611, w1613) -> (w1610:string[])
                  }
                }
                frame True {
                  w1626 = string[] []
                  n458 = for {
                    tunnel: w1627 -> [w1667] mode=indexing
                    tunnel: [w1670] -> w1635
                    tunnel: w1634 -> [w1668]
                    tunnel: [w1644] -> w1632 mode=indexing
                    tunnel: [w1641] -> w1631 mode=indexing
                    tunnel: [w1647] -> w1633 mode=indexing
                    tunnel: [w1638] -> w1630 mode=indexing
                    tunnel: w1629 -> [w1651]
                    tunnel: [w1650] -> w1628
                    shift-right: [w1646] -> w1622
                    shift-left: w1626 -> [w1645]
                    shift-right: [w1642] -> w1623
                    shift-left: w1626 -> [w1643]
                    shift-right: [w1639] -> w1624
                    shift-left: w1626 -> [w1640]
                    shift-right: [w1637] -> w1625
                    shift-left: w1626 -> [w1636]
                    w1649 = FALSE ("Log (T)")
                    w1664 = u16 0 items=["Voltage", "Current"] ("Source Mode  (0: Voltage)")
                    n459 = call "Ke2400 Configure Output.vi"("Source Mode  (0: Voltage)"=w1664, "error in (no error)"=w1651, "Compliance  Level (0.1)"=0.1, "Output Level (0)"=w1667, "VISA resource name"=w1668) -> ("error out"=w1674:errorcluster, "VISA resource name out"=w1672:refnum<visa-resource-name>)  [unwired: 5 in]
                    n460 = Number To Fractional String(number=w1667) -> (F-format string=w1666:string)  [unwired: 3 in]
                    n461 = call "Ke2400 Enable.vi"("error in (no error)"=w1674, "ON/OFF"=TRUE ("Enable Output (T: Enable)"), "VISA resource name"=w1672) -> ("error out"=w1675:errorcluster, "VISA resource name out"=w1670:refnum<visa-resource-name>)  [unwired: 7 in]
                    n462 = call "Delay.vi"("milliseconds to wait"=u32 10, "error in (no error)"=w1675) -> ("error out"=w1663:errorcluster)  [unwired: 9 in]
                    n463 = call "WS1050 AD7747 READ 36 DUT.vi"("error in"=w1663, "Log (T)"=w1649, "DUT Mask Mode (All)"=WSVCAP_SHL_I2C_DUT_Mask_Mode_Enum."C1") -> ("error out"=w1660:errorcluster, "AD7747 Values"=w1662:string[][])  [unwired: 7 in]
                    n464 = for {
                      tunnel: w1662 -> [w1686] mode=indexing
                      tunnel: [w1687] -> w1644 mode=indexing
                      tunnel: w1660 -> [w1685]
                      tunnel: [w1685] -> w1659
                      n465 = Index Array(array=w1686, index=1) -> (element=w1687:string)
                    }
                    n466 = Build Array (concatenate)(w1643, w1644) -> (w1642:string[])
                    n467 = call "WS1050 AD7747 READ 36 DUT.vi"("error in"=w1659, "Log (T)"=w1649, "DUT Mask Mode (All)"=WSVCAP_SHL_I2C_DUT_Mask_Mode_Enum."C2") -> ("error out"=w1657:errorcluster, "AD7747 Values"=w1656:string[][])  [unwired: 7 in]
                    n468 = for {
                      tunnel: w1656 -> [w1681] mode=indexing
                      tunnel: [w1682] -> w1641 mode=indexing
                      tunnel: w1657 -> [w1680]
                      tunnel: [w1680] -> w1655
                      n469 = Index Array(array=w1681, index=3) -> (element=w1682:string)
                    }
                    n470 = local write "STATUS"("VSA Testing...." ("STATUS")) -> ()
                    n471 = Build Array (concatenate)(w1640, w1641) -> (w1639:string[])
                    n472 = call "WS1050 AD7747 READ 36 DUT.vi"("error in"=w1655, "Log (T)"=w1649, "DUT Mask Mode (All)"=WSVCAP_SHL_I2C_DUT_Mask_Mode_Enum."C3") -> ("error out"=w1653:errorcluster, "AD7747 Values"=w1652:string[][])  [unwired: 7 in]
                    n473 = for {
                      tunnel: w1652 -> [w1677] mode=indexing
                      tunnel: [w1678] -> w1638 mode=indexing
                      tunnel: w1653 -> [w1676]
                      tunnel: [w1676] -> w1650
                      n474 = Index Array(array=w1677, index=5) -> (element=w1678:string)
                    }
                    n475 = for {
                      N: 36 -> [_]
                      tunnel: w1666 -> [w1684]
                      tunnel: [w1684] -> w1647 mode=indexing
                    }
                    n476 = Build Array (concatenate)(w1636, w1638) -> (w1637:string[])
                    n477 = Build Array (concatenate)(w1645, w1647) -> (w1646:string[])
                  }
                }
              }
              n478 = Transpose 2D Array(2D array=w1584) -> (transposed array=w1582:string[][])
              n479 = Transpose 2D Array(2D array=w1585) -> (transposed array=w1583:string[][])
              n480 = Transpose 2D Array(2D array=w1581) -> (transposed array=w1580:string[][])
              n481 = Transpose 2D Array(2D array=w1578) -> (transposed array=w1577:string[][])
              n482 = call "WS1050_VSA_Convert_Data.vi"("VSA_C3"=w1577, "error in (no error)"=w1579, "VSA_C2"=w1580, "VSA_C1"=w1582, "Voltage"=w1583) -> ("error out"=w1576:errorcluster, "VSA_V3"=→"VSA_V3":string[][], "VSA_V2"=→"VSA_V2":string[][], "VSA_V1"=→"VSA_V1":string[][])  [unwired: 3 in]
              n483 = case shown="True" w1563 {
                tunnel: w1588 -> [w1698 w1704]
                tunnel: [w1698 w1703] -> w1562
                tunnel: w1576 -> [w1697 w1702]
                tunnel: [w1697 w1699] -> w1587
                frame False {
                }
                frame True {
                  w1700 = u16 0 items=["Voltage", "Current"] ("Source Mode  (0: Voltage)")
                  n484 = call "Ke2400 Configure Output.vi"("Source Mode  (0: Voltage)"=w1700, "error in (no error)"=w1702, "Output Level (0)"=0.0, "VISA resource name"=w1704) -> ("error out"=w1699:errorcluster, "VISA resource name out"=w1703:refnum<visa-resource-name>)  [unwired: 6 in]
                }
              }
              n485 = call "Delay.vi"("milliseconds to wait"=u32 50, "error in (no error)"=w1587) -> ("error out"=w1565:errorcluster)  [unwired: 9 in]
              n486 = flat-sequence {
                tunnel: w1565 -> [w1598]
                tunnel: [w1597] -> w1566
                tunnel: [w1596] -> w1564
                tunnel: w1565 -> [w1596]
                tunnel: w1560 -> [w1595]
                tunnel: [w1595] -> w1559
                tunnel: w1556 -> [w1594]
                tunnel: w1555 -> [w1593]
                tunnel: w1554 -> [w1592]
                tunnel: w1553 -> [w1591]
                tunnel: w1552 -> [w1590]
                tunnel: [w1589] -> w1551
                frame #0 {
                  n487 = Build Array (concatenate)(w1593, w1594, w1592, w1591, w1590) -> (w1589:string[])
                  n488 = Select(t=WS105x_Run_Sequences."Save Data" ("WS105x Run Sequences"), s=w1598, f=WS105x_Run_Sequences."HS CHK" ("WS105x Run Sequences")) -> (s? t:f=w1597:T4)
                }
              }
            }
            frame "HS CHK" {
              n489 = for {
                tunnel: w1720 -> [w1737] mode=indexing
                tunnel: [w1736] -> w1719 mode=indexing
                tunnel: [w1735] -> w1717
                tunnel: w1718 -> [w1735]
                i -> [w1738]
                n490 = Index Array(array=w1737, index=w1738) -> (element=w1736:string)
              }
              n491 = case shown="False" w1726 {
                tunnel: w1724 -> [w1751 _]
                tunnel: w1717 -> [w1750 w1756]
                tunnel: [w1749 w1756] -> w1715
                tunnel: [w1745 w1755] -> w1707
                tunnel: [w1744 w1755] -> w1708
                tunnel: w1725 -> [w1743 _]
                tunnel: w1723 -> [w1742 _]
                tunnel: w1722 -> [w1741 _]
                tunnel: w1721 -> [w1740 _]
                tunnel: w1719 -> [w1739 _]
                frame False {
                  n492 = call "WS1050_36DUT_Handshake Check R1_Record All Regs Ver1.0.vi"("file path (use dialog)"=w1751, "Reg1_Bit Cntrl"="Reg1_Bit Cntrl", "File Name"=w1740, "SN"=w1739, "Loop"=w1743, "error"=w1750, "Lot #"=w1742, "Wafer #"=w1741) -> ("Pass/Fail"=→"EFuse Readback Status":bool[], "EFuse Read back"=w1744:string[], "Status"=w1745:string[], "error out"=w1749:errorcluster)  [unwired: 6 in, 2 out]
                  n493 = case shown="1, Default" w1743 {
                    tunnel: w1744 -> [w1752 w1753]
                    frame 0 {
                      "EFuse RB T0" <- w1752
                    }
                    frame 1, Default {
                      "Current EFuse Read back" <- w1753
                    }
                  }
                  n494 = local write "STATUS"("Hand Shake & EFuse Readback...." ("STATUS")) -> ()
                }
                frame True {
                  n495 = for {
                    N: 36 -> [_]
                    tunnel: [""] -> w1755 mode=indexing
                  }
                }
              }
              n496 = flat-sequence {
                tunnel: [w1732] -> w1716
                tunnel: w1715 -> [w1731]
                tunnel: [w1731] -> w1714
                tunnel: w1709 -> [w1730]
                tunnel: w1708 -> [w1729]
                tunnel: w1707 -> [w1728]
                tunnel: [w1727] -> w1706
                frame #0 {
                  n497 = Build Array (concatenate)(w1730, w1729, w1728) -> (w1727:string[])
                  n498 = Select(t=WS105x_Run_Sequences."Save Data" ("WS105x Run Sequences"), s=w1731, f=WS105x_Run_Sequences."Save Data" ("WS105x Run Sequences")) -> (s? t:f=w1732:T4)
                }
              }
            }
            frame "Save Data" {
              n499 = Path To String(path=w1767) -> (string=w1770:string)
              n500 = Concatenate Strings(w1770, "\\" ("string"), w1763, "_Multi Socket Data.csv" ("string")) -> (w1766:string)
              n501 = flat-sequence {
                tunnel: w1779 -> [w1791]
                tunnel: w1767 -> [w1790]
                tunnel: [w1789] -> w1778
                tunnel: w1766 -> [w1788]
                tunnel: [w1788] -> w1765
                tunnel: w1764 -> [w1786]
                tunnel: w1763 -> [w1787]
                tunnel: w1762 -> [w1785]
                tunnel: w1765 -> [w1793]
                tunnel: "Plot Delta Cmin" -> [w1794]
                tunnel: w1778 -> [w1795]
                tunnel: [w1792] -> w1761
                tunnel: [w1813] -> w1775
                tunnel: w1761 -> [w1813]
                tunnel: w1760 -> [w1814]
                tunnel: [w1812] -> w1759
                frame #0 {
                  n502 = local write "STATUS"("Save Data...." ("STATUS")) -> ()
                  n503 = call "WS1050_36 DUT CPCV SData Ver1.2.vi"("All Data Out"=w1786, "error in"=w1791, "File Name"=w1787, "Cap Header"=w1785, "TMN DC\\CAP Data Log File Path"=w1790) -> ("error out"=w1789:errorcluster)  [unwired: 5 in]
                }
                frame #1 {
                  n504 = case shown="True" w1794 {
                    tunnel: w1795 -> [w1796 w1810]
                    tunnel: [w1796 w1806] -> w1792
                    tunnel: w1793 -> [_ w1797]
                    frame False {
                    }
                    frame True {
                      n505 = call "Delay.vi"("milliseconds to wait"=u32 50, "error in (no error)"=w1810) -> ("error out"=w1809:errorcluster)  [unwired: 9 in]
                      n506 = String To Path(string=w1797) -> (path=w1802:path)
                      n507 = call "36DUT Plot From Spread Sheet.vi"("Plot"="Plot", "error in (no error)"=w1809, "Bank"="Bank C1", "file path (dialog if empty)"=w1802) -> ("error out"=w1804:errorcluster, "Delta C_Min Plot"=→"Min Plot_1":dbl[][])  [unwired: 6 in]
                      n508 = call "36DUT Plot From Spread Sheet.vi"("Plot"="Plot", "error in (no error)"=w1804, "Bank"="Bank C2", "file path (dialog if empty)"=w1802) -> ("error out"=w1805:errorcluster, "Delta C_Min Plot"=→"Min Plot_2":dbl[][])  [unwired: 6 in]
                      n509 = call "36DUT Plot From Spread Sheet.vi"("Plot"="Plot", "error in (no error)"=w1805, "Bank"="Bank C3", "file path (dialog if empty)"=w1802) -> ("error out"=w1806:errorcluster, "Delta C_Min Plot"=→"Min Plot_3":dbl[][])  [unwired: 6 in]
                    }
                  }
                }
                frame #2 {
                  n510 = Greater Or Equal?(x=w1814, y="Set HD/Cycle \nto Complete") -> (x >= y?=w1812:bool)
                }
              }
              n511 = local read "No of HD/Cycle\nCompleted"() -> (w1760:u64)
              n512 = flat-sequence {
                tunnel: [w1781] -> w1776
                tunnel: w1759 -> [w1780]
                frame #0 {
                  n513 = Select(t=WS105x_Run_Sequences."Idle..." ("WS105x Run Sequences"), s=w1780, f=WS105x_Run_Sequences."CPV SWPT" ("WS105x Run Sequences")) -> (s? t:f=w1781:T4)
                }
              }
              "All Data Out" <- w1764
            }
            frame "CPV SWPT" {
              n514 = case shown="False" "Auto\nMan" {
                tunnel: [w1833 w1840] -> w1826
                tunnel: "Start" -> [_ w1839]
                tunnel: "Step" -> [_ w1838]
                tunnel: "Stop" -> [_ w1837]
                tunnel: w1825 -> [w1834 w1836]
                tunnel: [w1834 w1835] -> w1827
                tunnel: "Manual Setting\nFor RP CP CV" -> [w1833 _]
                frame False {
                }
                frame True {
                  n515 = call "Generate RP for CP CV Sweep.vi"("Start"=w1839, "Step"=w1838, "Stop"=w1837, "error in (no error)"=w1836) -> ("RP for CP CV"=w1840:i64[], "error out"=w1835:errorcluster)  [unwired: 10 in]
                }
              }
              "RP for CP CV" <- w1826
              n516 = case shown="True" "CP CV \nSweep" {
                tunnel: w1827 -> [w1843 w1857]
                tunnel: [w1842 w1849] -> w1822
                tunnel: w1824 -> [_ w1852]
                tunnel: w1826 -> [_ w1851]
                tunnel: [w1841 w1848] -> w1817
                frame False {
                  n517 = flat-sequence {
                    tunnel: [w1845] -> w1841
                    tunnel: w1843 -> [w1844]
                    tunnel: [w1844] -> w1842
                    frame #0 {
                      n518 = Select(t=WS105x_Run_Sequences."Idle..." ("WS105x Run Sequences"), s=w1844, f=WS105x_Run_Sequences."Vdd" ("WS105x Run Sequences")) -> (s? t:f=w1845:T4)
                    }
                  }
                }
                frame True {
                  n519 = call "Read Point CP CV Sweep.vi"("error in"=w1857, "Set Point for\nCV CV Sweep"=w1851) -> ("error Out"=w1856:errorcluster, "Last Number"=w1853:u64, "Ind"=w1855:bool)  [unwired: 5 in, 2 out]
                  n520 = Number To Exponential String(number=w1853) -> (E-format string=w1854:string)  [unwired: 3 in]
                  n521 = case shown="True" w1855 {
                    tunnel: w1856 -> [w1862 w1871]
                    tunnel: [w1862 w1870] -> w1850
                    tunnel: w1854 -> [_ w1869]
                    tunnel: w1852 -> [_ w1863]
                    frame False {
                    }
                    frame True {
                      n522 = call "WS1050 36 DUT CP CV Sweep F12_B1_Ver1.2.vi"("error in (no error)"=w1871, "File Name"=w1863, "HD/Cycles Completed"=w1869) -> ("Plot_1"=→"CP CV Sweep C1":dbl[][], "Plot_2"=→"CP CV Sweep C2":dbl[][], "Plot_3"=→"CP CV Sweep C3":dbl[][], "CP Voltage"=→"LP CP Voltage":string, "error out"=w1870:errorcluster)  [unwired: 14 in, 6 out]
                      n523 = local write "STATUS"("CP CV Sweep..." ("STATUS")) -> ()
                    }
                  }
                  n524 = flat-sequence {
                    tunnel: [w1859] -> w1848
                    tunnel: w1850 -> [w1858]
                    tunnel: [w1858] -> w1849
                    frame #0 {
                      n525 = Select(t=WS105x_Run_Sequences."Idle..." ("WS105x Run Sequences"), s=w1858, f=WS105x_Run_Sequences."CPV Data" ("WS105x Run Sequences")) -> (s? t:f=w1859:T4)
                    }
                  }
                }
              }
            }
            frame "CPV Data" {
              n526 = flat-sequence {
                tunnel: [w1879] -> w1873
                tunnel: w1872 -> [w1881]
                frame #0 {
                  n527 = Select(t=WS105x_Run_Sequences."Idle..." ("WS105x Run Sequences"), s=w1881, f=WS105x_Run_Sequences."Vdd" ("WS105x Run Sequences")) -> (s? t:f=w1879:T4)
                }
              }
            }
            frame "Idle...", Default {
              n528 = flat-sequence {
                tunnel: [w1892] -> w1888
                tunnel: w1884 -> [w1889]
                frame #0 {
                  n529 = Select(t=WS105x_Run_Sequences."Vdd" ("WS105x Run Sequences"), s=w1889, f=WS105x_Run_Sequences."Vdd" ("WS105x Run Sequences")) -> (s? t:f=w1892:T4)
                }
              }
            }
          }
          n530 = Increment(x=w337) -> (x+1=→"Loop \ncompleted":i32)
          n531 = Unbundle By Name(w360) -> ("status"=w331:bool)
          n532 = Compound Arithmetic op=OR(w331, w330) -> (w359:bool)
        }
      }
      frame True {
      }
    }
    n533 = Unbundle By Name(w112) -> ("status"=w111:bool)
    n534 = Compound Arithmetic op=OR(w111, w78) -> (w113:bool)
    "STATUS" <- "Idle...." ("STATUS")
  }
  n535 = local write "stop During HD/Cycles"(w9) -> ()
  n536 = local write "stop"(w9) -> ()
  n537 = case shown="True" w14 {
    tunnel: [w1897 w1900] -> w11
    tunnel: w12 -> [w1897 w1899]
    frame False {
    }
    frame True {
      n538 = local write "Online"(FALSE ("Online")) -> ()
      n539 = call "WSVCAP SHL Host TL Close.vi"("error in"=w1899) -> ("error out"=w1900:errorcluster)  [unwired: 14 in]
    }
  }
  n540 = VISA Write(VISA resource name=w10, write buffer="SOUR:FUNC VOLT;VOLT:MODE FIX;RANG 100;LEV 0.0;:SENS:FUNC \"CURR\";CURR:PROT 60E-3;RANG 100E-3;:OUTP OFF", error in (no error)=w12) -> (VISA resource name out=w5:refnum<visa-resource-name>, error out=w8:errorcluster)  [unwired: 1 out]
  n541 = VISA Write(VISA resource name=w13, write buffer=":INST:NSEL 1; :VOLT 0.000000;:OUTP 1;", error in (no error)=w12) -> (VISA resource name out=w3:refnum<visa-resource-name>, error out=w2:errorcluster)  [unwired: 1 out]
  n542 = Build Array(w5, w4, w3) -> (w1:refnum<visa-resource-name>[])
  n543 = Merge Errors(w11, w8, w2) -> (w7:errorcluster)
  n544 = for {
    tunnel: w7 -> [w1903]
    tunnel: [w1902] -> w6
    tunnel: w1 -> [w1901] mode=indexing
    n545 = VISA Close(VISA resource name=w1901, error in (no error)=w1903) -> (error out=w1902:errorcluster)
  }
  "error out" <- w6
